vi "HostHoppingScan_v2_BoostedMultiRegion.vi"() -> ()   [LabVIEW 2024]
uses:
  <vilib>/Analysis/6fits.llb/Curve Fitting Criteria.ctl
  <vilib>/FPGAPlugInAG/USB-7845R OEM/niLvFpga_Open_USB-7845R OEM.vi
  <vilib>/rvi/interface/common/dynamic/niFpgaDynamicAddResources.vi
  <vilib>/Utility/error.llb/Error Cluster From Error Code.vi
  <vilib>/rvi/errors/niLvFpgaAdjustHostInterfaceError.vi
  <vilib>/rvi/interface/common/niFpgaWaitOnOcc.vi
  <vilib>/FPGAPlugInAG/Dynamic/niLvFpga_Close_Dynamic.vi
  <vilib>/rvi/interface/nirviOpenFPGA/nirviOpenFPGA.xnode
  FPGA Bitfiles/hoppingsicmv2_FPGATarget_FPGAHoppingScanB_lvkcmxVGkic.lvbitx
  <vilib>/rvi/interface/nirviMethod/nirviMethod.xnode
  <vilib>/rvi/interface/nirviReadWriteControl/nirviReadWriteControl.xnode
  <vilib>/rvi/interface/nirviCloseFPGA/nirviCloseFPGA.xnode
  NiFpgaLv.dll
  <vilib>/rvi/interface/Simulation/niFpgaSimulationCallBeginRW.vi
  <vilib>/rvi/errors/niLvFpgaMergeErrorWithErrorCode.vi
  <vilib>/FPGAPlugInAG/Dynamic/niLvFpga_ReadFifo_Dynamic.vi
  <vilib>/FPGAPlugInAG/Dynamic/niLvFpga_WriteFifo_Dynamic.vi
  <vilib>/Analysis/NI_AALPro.lvlib
  <vilib>/FPGAPlugInAG/Dynamic/niLvFpga_ConfigureFifo_Dynamic.vi
panel:
  out "RegionScanning":string
  in  "Auto Image \nSegmentation?":bool
  out "Adapted_YOffset um":dbl format="%#_13g"
  out "Adapted_XOffset um":dbl format="%#_13g"
  out "Adapted_YNum":i32
  out "Adapted_XNum":i32
  in  "Scanning Settings":T1(tab)
  in  "Retract (edge) um":dbl format="%#_13g"
  in  "FrameNum":u32
  in  "XNum":i32
  in  "YNum":i32
  in  "FF_Threshold %":dbl format="%#_13g"
  in  "XStepSize um":dbl format="%#_13g"
  in  "YStepSize um":dbl format="%#_13g"
  in  "YOffset um":dbl format="%#_13g"
  in  "XOffset um":dbl format="%#_13g"
  in  "Retract (flat) um":dbl format="%#_13g"
  in  "RetRate um/s":dbl format="%#_13g"
  in  "FF_AppRate um/s":dbl format="%#_13g"
  in  "NF_AppRate um/s":dbl format="%#_13g"
  in  "Pressure kPa":dbl format="%#_13g"
  in  "NF_Threshold %":dbl format="%#_13g"
  in  "Turning Distance um":dbl format="%#_13g"
  in  "CoordCalThreshold %":dbl format="%#_13g"
  in  "CoordCalRetract um":dbl format="%#_13g"
  in  "YCoordCalEnd um":dbl format="%#_13g"
  in  "XCoordCalEnd um":dbl format="%#_13g"
  in  "YCoordCalBegin um":dbl format="%#_13g"
  in  "XCoordCalBegin um":dbl format="%#_13g"
  in  "CoordCalAppRate um/s":dbl format="%#_13g"
  in  "CoordCalRetRate um/s":dbl format="%#_13g"
  in  "ScanMode":i32(knob) min=0 max=3 scale=0.0..3.0
  out "Signal Size":i32
  out "Done?":bool
  out "HTT_Buffer_Write":u32
  out "Scanned Points":i32
  in  "stop":bool
  in  "Notes":string
  in  "GraphTab":T2(tab)
  out "Topography":dbl[][](graph)
  out "Retract Map":dbl[][](graph)
  out "IZCurve":cluster{dbl[], dbl[]}(graph)
  out "Pressure Slope Map":dbl[][](graph)
  out "FPGA_Host_Buf_Depth":u32
  # "Calibrated Scan\n(New Calibration)"
  # "Calibrated Scan\n(Last Calibration)"
  # "Normal Scan"
  # "Background\nSubstrate Scan"
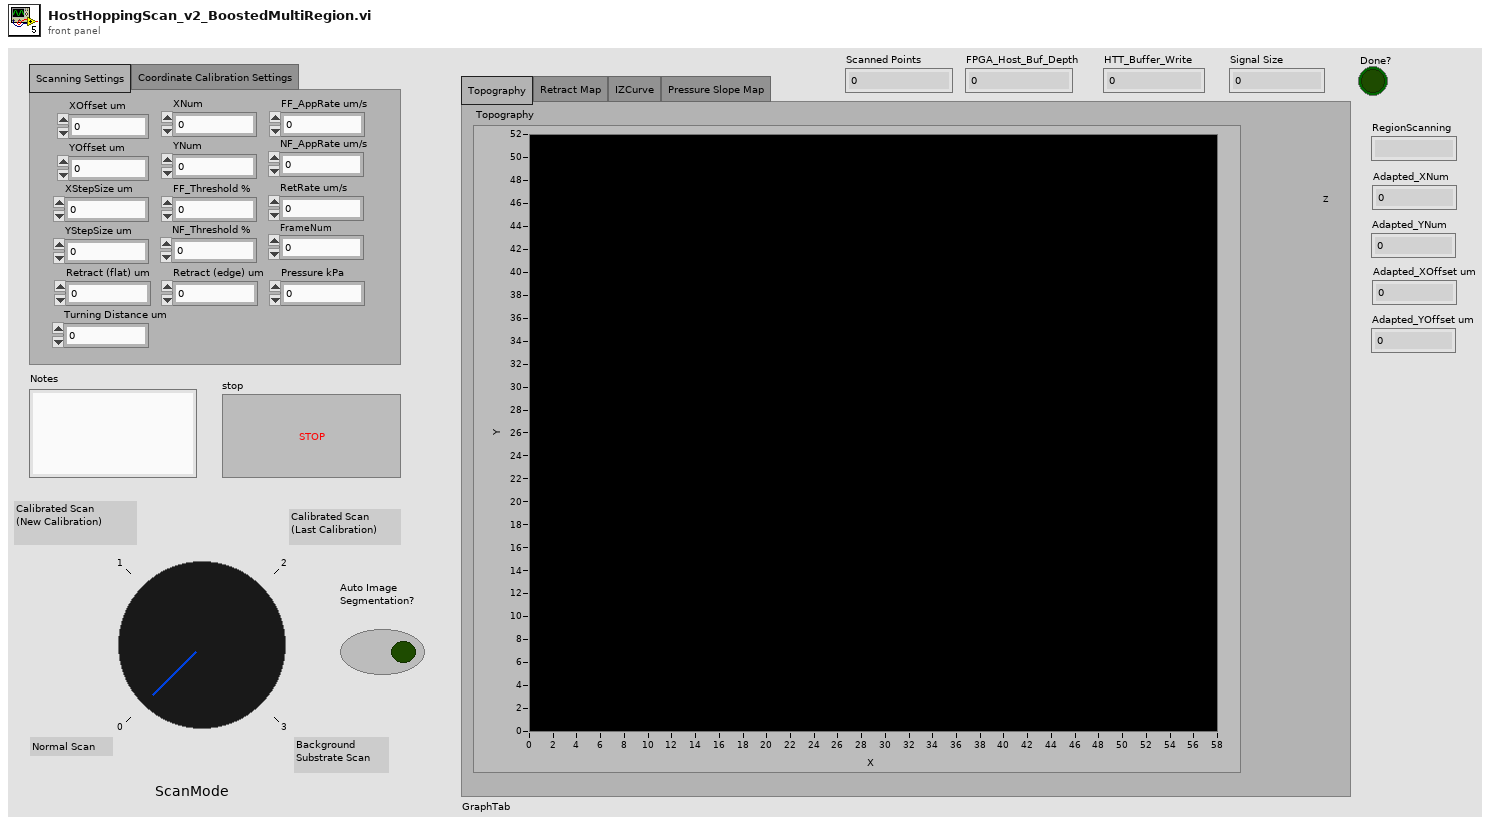
[diagram p1: front panel]
types:
  T1 = enum32{"Scanning Settings", "Coordinate Calibration Settings"}
  T2 = enum32{"Topography", "Retract Map", "IZCurve", "Pressure Slope Map"}
  T3 = typedef "NI_AALPro.lvlib/Curve Fitting Criteria.ctl" = u16
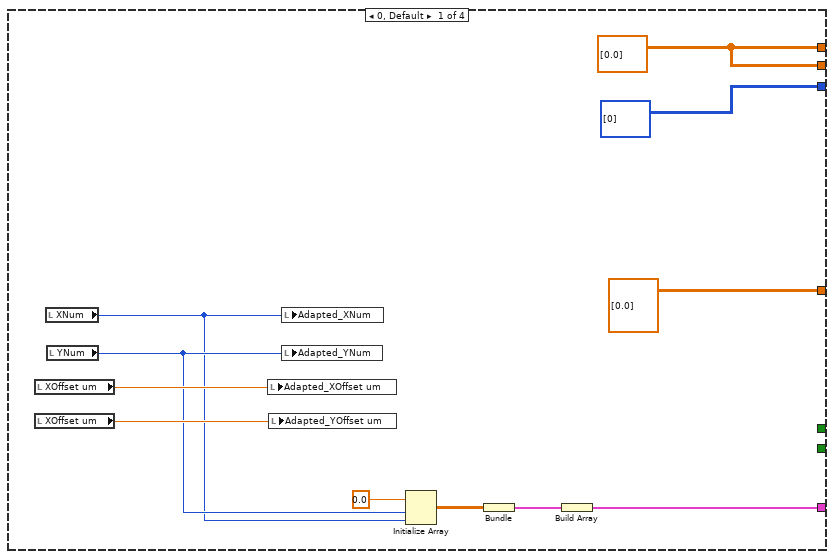
[diagram p3: hidden frame]
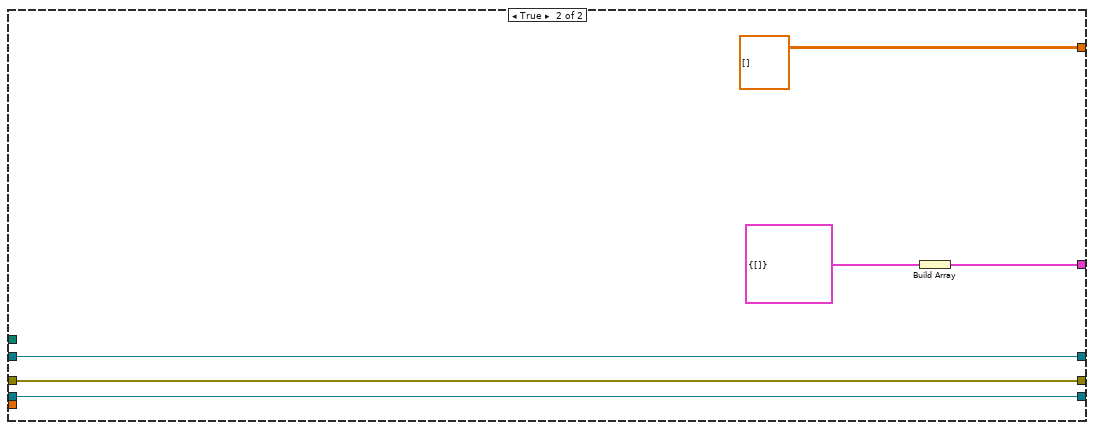
[diagram p4: hidden frame]
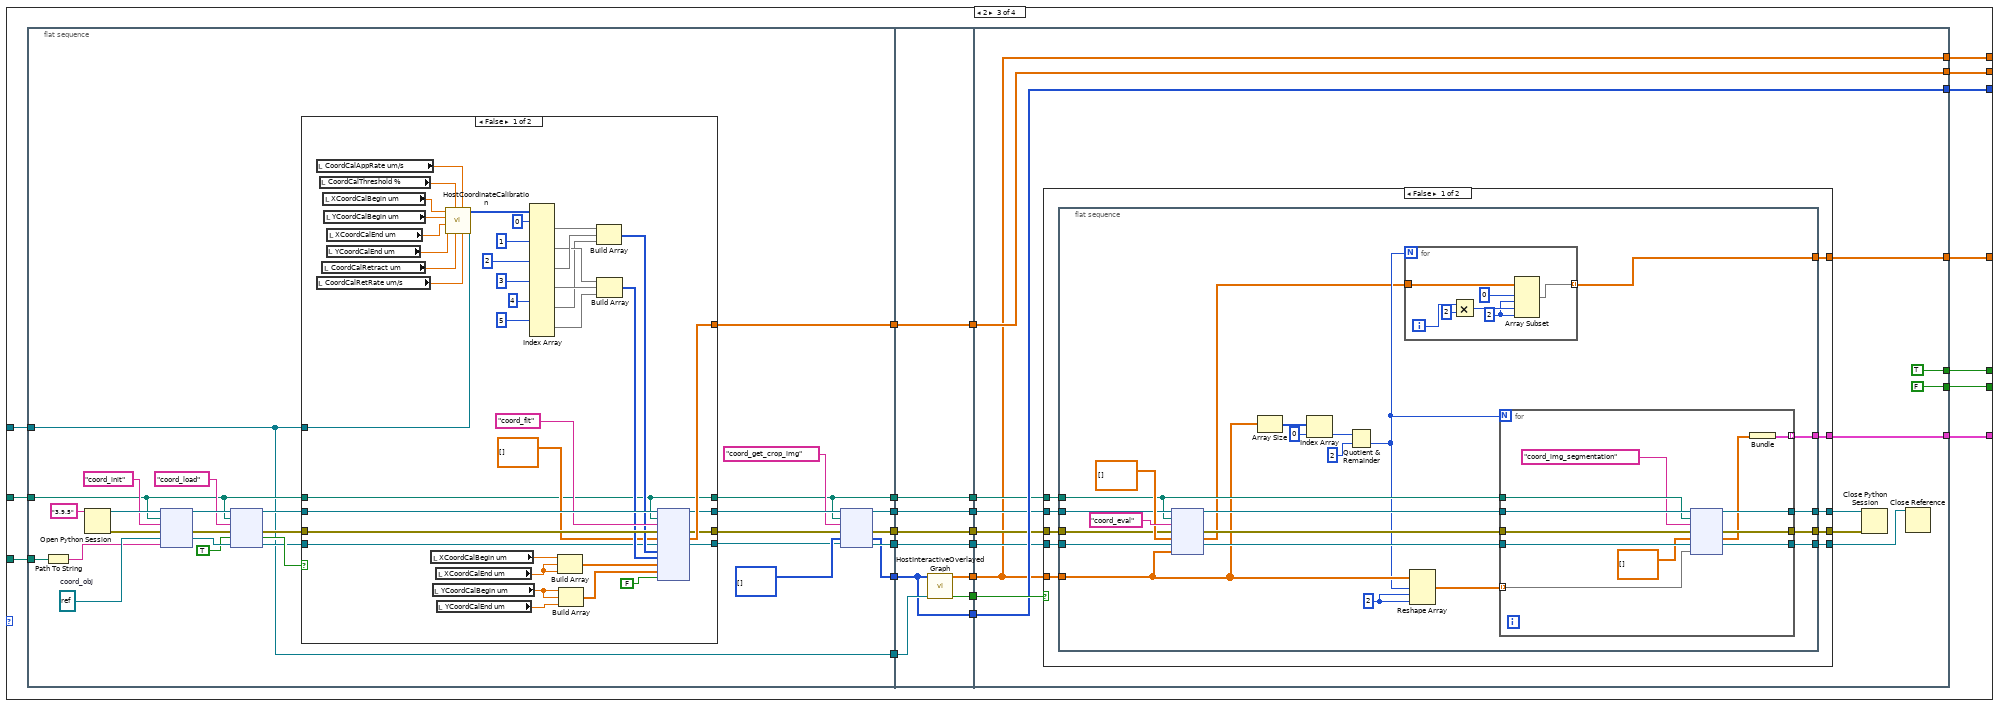
[diagram p5: hidden frame]
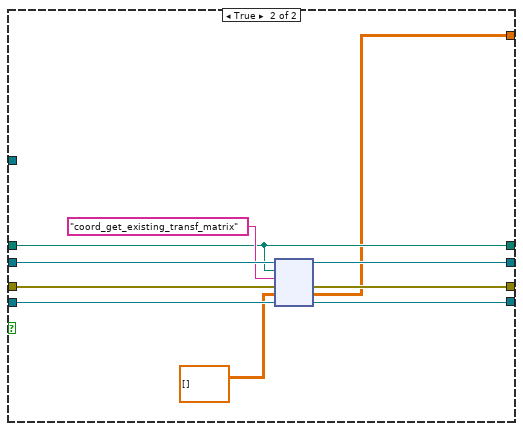
[diagram p6: hidden frame]
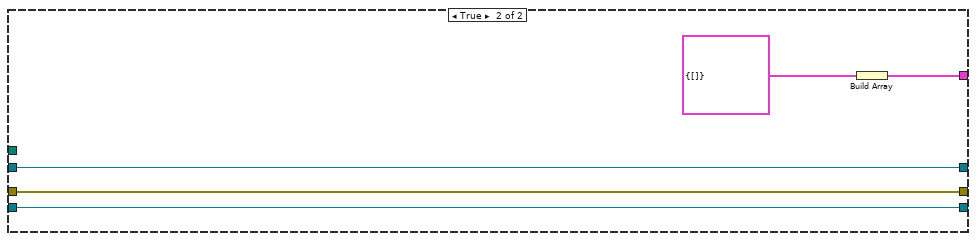
[diagram p7: hidden frame]
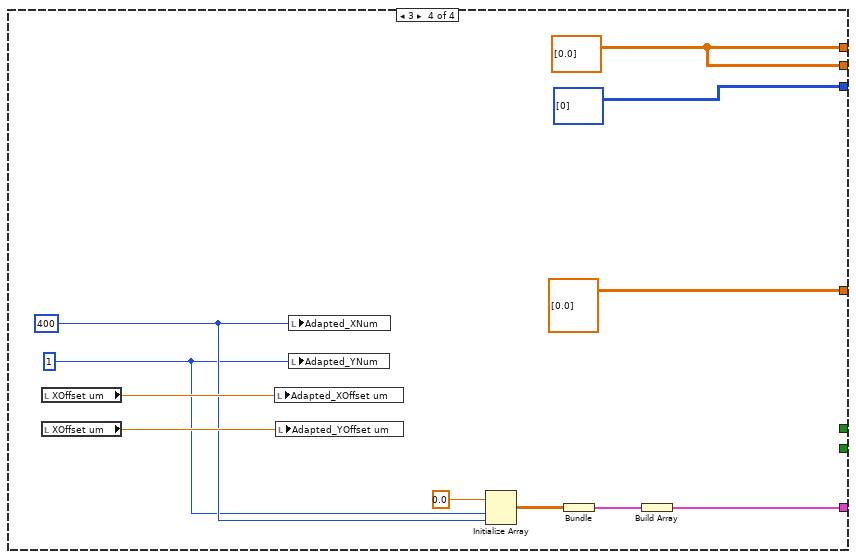
[diagram p8: hidden frame]
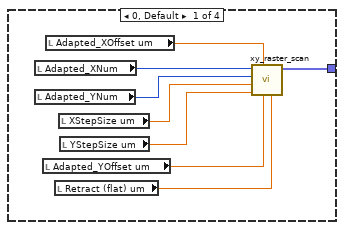
[diagram p14: hidden frame]
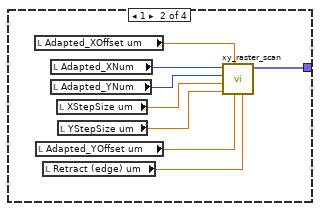
[diagram p15: hidden frame]
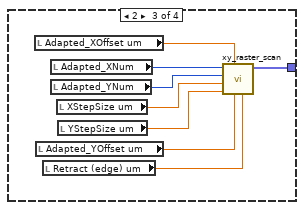
[diagram p16: hidden frame]
diagram:
  n1 = flat-sequence {
    tunnel: [w4] -> w2
    tunnel: w2 -> [w30]
    tunnel: [w27] -> w1
    tunnel: w1 -> [w1444]
    frame #0 {
      n2 = Obtain Queue(max queue size (-1, unlimited)=64, name (unnamed)="stop_sign", element data type=FALSE) -> (queue out=w4:refnum<queue>)  [unwired: 2 in, 2 out]
    }
    frame #1 {
      n3 = flat-sequence {
        tunnel: [w52] -> w31
        tunnel: w30 -> [w52]
        tunnel: w31 -> [w58]
        tunnel: [w58] -> w25
        tunnel: [w54] -> w24
        tunnel: [w107] -> w22
        tunnel: [w108] -> w21
        tunnel: [w109] -> w20
        tunnel: [w110] -> w19
        tunnel: [w111] -> w18
        tunnel: [w74] -> w17
        tunnel: w24 -> [w92]
        tunnel: w25 -> [w74]
        tunnel: [w72] -> w16
        tunnel: [w499] -> w39
        tunnel: [w497] -> w38
        tunnel: [w496] -> w37
        tunnel: [w498] -> w36
        tunnel: [w501] -> w29
        tunnel: w22 -> [w496]
        tunnel: w21 -> [w497]
        tunnel: w20 -> [w499]
        tunnel: w19 -> [w498]
        tunnel: w18 -> [w490]
        tunnel: [w490] -> w23
        tunnel: w17 -> [w494]
        tunnel: w16 -> [w491]
        tunnel: [w491] -> w15
        tunnel: [w489] -> w14
        tunnel: w39 -> [w526]
        tunnel: w38 -> [w525]
        tunnel: w37 -> [w524]
        tunnel: [w522] -> w35
        tunnel: [w521] -> w34
        tunnel: [w520] -> w33
        tunnel: [w519] -> w32
        tunnel: w36 -> [w523]
        tunnel: w29 -> [w518]
        tunnel: [w517] -> w28
        tunnel: w23 -> [w516]
        tunnel: w15 -> [w515]
        tunnel: w14 -> [w514]
        tunnel: [w514] -> w13
        tunnel: [w513] -> w12
        tunnel: [w512] -> w11
        tunnel: [w511] -> w10
        tunnel: [w510] -> w9
        tunnel: [w509] -> w8
        tunnel: [w508] -> w7
        tunnel: w35 -> [w1430]
        tunnel: w34 -> [w1436]
        tunnel: w33 -> [w1435]
        tunnel: w32 -> [w1434]
        tunnel: w28 -> [w1428]
        tunnel: [w1428] -> w26
        tunnel: w13 -> [w1418]
        tunnel: w12 -> [w1417]
        tunnel: w11 -> [w1416]
        tunnel: w10 -> [w1415]
        tunnel: w9 -> [w1414]
        tunnel: w8 -> [w1413]
        tunnel: w7 -> [w1412]
        tunnel: [w1443] -> w27
        tunnel: w26 -> [w1443]
        frame #0 {
          n4 = Wait (ms)(milliseconds to wait=u32 100) -> ()  [unwired: 1 out]
          "Done?" <- FALSE ("Done?")
          "Adapted_XNum" <- "XNum"
          "Adapted_YNum" <- "YNum"
          "Adapted_XOffset um" <- "XStepSize um"
          "Adapted_YOffset um" <- "YStepSize um"
        }
        frame #1 {
          n5 = call "File Dialog"("prompt"="Choose a path to save scanning image data files") -> ("selected path"=w54:path, "cancelled"=w56:bool, "error out"=w55:errorcluster)  [unwired: 11 in, 1 out]
          n6 = Stop(stop? (T)=w56) -> ()
          n7 = call <vilib>:"Clear Errors.vi"("error in (no error)"=w55) -> ()  [unwired: 5 in, 2 out]
        }
        frame #2 {
          w73 = refnum<k38> refnum  # db_obj
          # "coordinate calibration"
          # "use python to save data this time"
          n8 = Path To String(path=w92) -> (string=w106:string)
          n9 = local read "ScanMode"() -> (w75:i32)
          n10 = Get Queue Status(queue=w74) -> (# elements in queue=w91:i32)  [unwired: 2 in, 7 out]
          n11 = Concatenate Strings(w106, "_data.db" ("string")) -> (w105:string)
          n12 = Current VI's Path() -> (path=w97:path)
          n13 = Less Or Equal To 0?(x=w91) -> (x <= 0?=w90:bool)
          n14 = String To Path(string=w105) -> (path=w103:path)
          n15 = Strip Path(path=w97) -> (stripped path=w85:path)  [unwired: 1 out]
          n16 = call <vilib>:"Check if File or Folder Exists.vi"("path"=w103) -> ("file or folder exists?"=w104:bool)  [unwired: 8 in, 2 out]
          n17 = Build Path(base path=w85, name or relative path=path "py/coord_transform.py") -> (appended path=w87:path)
          n18 = Build Path(base path=w85, name or relative path=path "coordinate_calibration/tmp_calibrated_coord") -> (appended path=w84:path)
          n19 = Select(t=w75, s=w90, f=0 ("t")) -> (s? t:f=w89:i32)
          n20 = Build Path(base path=w85, name or relative path=path "py/data_db_arrangement_boosted_multi_region.py") -> (appended path=w110:path)
          n21 = case shown="1" w89 {
            tunnel: w87 -> [_ w145 w313 _]
            tunnel: w84 -> [_ w147 w312 _]
            tunnel: w74 -> [_ w146 w311 _]
            tunnel: [w120 w144 w290 w477] -> w111
            tunnel: [i32[][] [[0]] w143 w292 i32[][] [[0]]] -> w60
            tunnel: [w119 w142 w291 w485] -> w61
            tunnel: [w119 w141 w293 w485] -> w62
            tunnel: [_ w140 w294 _] -> w63
            tunnel: [_ w139 w295 _] -> w64
            tunnel: [dbl[][][] [[[0.0]]] ("OutputRetractMap um") w123 w289 dbl[][][] [[[0.0]]] ("OutputRetractMap um")] -> w72
            frame 0, Default {
              w119 = dbl[][] [[0.0]] ("Output_Coord")
              n22 = local read "XOffset um"() -> (w122:dbl)
              n23 = local read "XOffset um"() -> (w121:dbl)
              n24 = local read "XNum"() -> (w112:i32)
              n25 = local read "YNum"() -> (w113:i32)
              n26 = local write "Adapted_XOffset um"(w122) -> ()
              n27 = local write "Adapted_YOffset um"(w121) -> ()
              n28 = local write "Adapted_XNum"(w112) -> ()
              n29 = local write "Adapted_YNum"(w113) -> ()
              n30 = Initialize Array(0.0, w113, w112) -> (w115:dbl[][])
              n31 = Bundle(w115) -> (w114:cluster{dbl[][]})  [unwired: 1 in]
              n32 = Build Array(w114) -> (w120:cluster{dbl[][]}[])
            }
            frame 1 {
              n33 = flat-sequence {
                tunnel: w147 -> [w196]
                tunnel: w146 -> [w149]
                tunnel: w145 -> [w152]
                tunnel: [w152] -> w129
                tunnel: [w160] -> w131
                tunnel: [w155] -> w133
                tunnel: [w154] -> w135
                tunnel: [w153] -> w136
                tunnel: [w150] -> w138
                tunnel: [w149] -> w127
                tunnel: w138 -> [w210]
                tunnel: [w210] -> w137
                tunnel: w136 -> [w202]
                tunnel: w135 -> [w209]
                tunnel: [w209] -> w134
                tunnel: w133 -> [w208]
                tunnel: [w208] -> w132
                tunnel: w131 -> [w207]
                tunnel: [w207] -> w130
                tunnel: w129 -> [w206]
                tunnel: [w206] -> w128
                tunnel: w127 -> [w205]
                tunnel: [w204] -> w126
                tunnel: [w203] -> w125
                tunnel: [w202] -> w124
                tunnel: [w222] -> w144
                tunnel: [w212] -> w143
                tunnel: [w214] -> w142
                tunnel: [w221] -> w141
                tunnel: [TRUE] -> w140
                tunnel: [FALSE] -> w139
                tunnel: w137 -> [w221]
                tunnel: w134 -> [w216]
                tunnel: w132 -> [w217]
                tunnel: w130 -> [w218]
                tunnel: w128 -> [w215]
                tunnel: w126 -> [w214]
                tunnel: w125 -> [w213]
                tunnel: w124 -> [w212]
                tunnel: [w211] -> w123
                frame #0 {
                  w197 = refnum<k38> refnum  # coord_obj
                  # "extended img bundle"
                  # "retracted img bundle"
                  n34 = Path To String(path=w196) -> (string=w195:string)
                  n35 = local read "CoordCalAppRate um/s"() -> (w189:dbl)
                  n36 = local read "CoordCalRetRate um/s"() -> (w187:dbl)
                  n37 = local read "CoordCalThreshold %"() -> (w190:dbl)
                  n38 = local read "CoordCalRetract um"() -> (w188:dbl)
                  n39 = local read "XCoordCalBegin um"() -> (w194:dbl)
                  n40 = local read "YCoordCalBegin um"() -> (w193:dbl)
                  n41 = local read "YCoordCalEnd um"() -> (w191:dbl)
                  n42 = local read "XCoordCalEnd um"() -> (w192:dbl)
                  n43 = Open Python Session(python version="3.9.5" ("Python version")) -> (session out=w200:refnum<k35>, error out=w199:errorcluster)  [unwired: 2 in]
                  n44 = node(w200, w152, "coord_init" ("Python version"), w199, w197, w195) -> (w174:refnum<k35>, w172:errorcluster, w173:refnum<k38>)  [unwired: 1 in, 2 out]
                  n45 = call "HostCoordinateCalibration.vi"("stop_sign_queue"=w149, "RetRate um/s"=w187, "AppRate um/s"=w189, "Retract um"=w188, "Threshold %"=w190, "YCalibrationEnd um"=w191, "XCalibrationEnd um"=w192, "YCalibrationOffset um"=w193, "XCalibrationOffset um"=w194) -> ("img_bundle"=w186:i32[][][])  [unwired: 2 in]
                  n46 = local read "XCoordCalBegin um"() -> (w169:dbl)
                  n47 = local read "YCoordCalBegin um"() -> (w166:dbl)
                  n48 = local read "XCoordCalEnd um"() -> (w168:dbl)
                  n49 = local read "YCoordCalEnd um"() -> (w167:dbl)
                  n50 = Index Array(array=w186, index (dim 0) #1=0 ("index (page)"), index (dim 0) #2=1 ("index (page)"), index (dim 0) #3=2 ("index (page)"), index (dim 0) #4=3 ("index (page)"), index (dim 0) #5=4 ("index (page)"), index (dim 0) #6=5 ("index (page)")) -> (element #1=w148:i32[][], element #2=w178:i32[][], element #3=w179:i32[][], element #4=w177:i32[][], element #5=w176:i32[][], element #6=w175:i32[][])  [unwired: 12 in]
                  n51 = Build Array(w169, w168, w168) -> (w165:dbl[])
                  n52 = Build Array(w166, w166, w167) -> (w164:dbl[])
                  n53 = Build Array(w148, w179, w176) -> (w171:i32[][][])
                  n54 = Build Array(w178, w177, w175) -> (w170:i32[][][])
                  n55 = node(w174, w152, "coord_fit" ("function name"), w172, dbl[][] [], w173, w171, w170, w165, w164, TRUE) -> (w161:refnum<k35>, w159:errorcluster, w150:dbl[][], w157:refnum<k38>)  [unwired: 5 in, 2 out]
                  n56 = node(w161, w152, "coord_get_crop_img" ("function name"), w159, i32[][] [], w157) -> (w160:refnum<k35>, w155:errorcluster, w153:i32[][], w154:refnum<k38>)  [unwired: 2 out]
                }
                frame #1 {
                  n57 = call "HostInteractiveOverlayedGraph.vi"("stop_sign_queue"=w205, "InputImg"=w202) -> ("Break"=w203:bool, "Output_Coord"=w204:dbl[][])  [unwired: 8 in]
                }
                frame #2 {
                  n58 = case shown="False" w213 {
                    tunnel: [w235 w288] -> w225
                    tunnel: [w234 w287] -> w224
                    tunnel: [w233 w286] -> w223
                    tunnel: [w227 w283] -> w222
                    tunnel: w214 -> [w232 _]
                    tunnel: w218 -> [w231 w288]
                    tunnel: w217 -> [w230 w287]
                    tunnel: w216 -> [w229 w286]
                    tunnel: w215 -> [w228 _]
                    tunnel: [w226 dbl[][][] [] ("OutputRetractMap um")] -> w211
                    frame False {
                      n59 = flat-sequence {
                        tunnel: [w245] -> w227
                        tunnel: [w255] -> w233
                        tunnel: [w256] -> w234
                        tunnel: [w257] -> w235
                        tunnel: w228 -> [w246]
                        tunnel: w229 -> [w252]
                        tunnel: w230 -> [w253]
                        tunnel: w231 -> [w254]
                        tunnel: w232 -> [w237]
                        tunnel: [w239] -> w226
                        frame #0 {
                          n60 = node(w254, w246, "coord_eval" ("function name"), w253, dbl[][] [], w252, w237) -> (w249:refnum<k35>, w248:errorcluster, w240:dbl[][], w247:refnum<k38>)  [unwired: 1 in, 2 out]
                          n61 = Array Size(array=w237) -> (size(s)=w244:i32[])
                          n62 = Index Array(array=w244, index=0) -> (element=w242:i32)
                          n63 = Quotient & Remainder(x=w242, y=2 ("index")) -> (floor(x/y)=w238:i32)  [unwired: 1 out]
                          n64 = for {
                            N: w238 -> [_]
                            tunnel: w237 -> [w263]
                            tunnel: [w258] -> w236 mode=indexing
                            i -> [w262]
                            n65 = Multiply(x=w262, y=2) -> (x*y=w260:i32)
                            n66 = Array Subset(array=w263, index (row)=w260, length (row)=2 ("length")) -> (w258:dbl[][])  [unwired: 2 in]
                          }
                          n67 = for {
                            N: w238 -> [_]
                            tunnel: w240 -> [w267]
                            tunnel: [w266] -> w239 mode=indexing
                            i -> [w264]
                            w268 = 2 ("length")
                            n68 = Multiply(x=2 ("y"), y=w264) -> (x*y=w270:i32)
                            n69 = Array Subset(array=w267, index (row)=0 ("index"), length (row)=w268, index (col)=w270, length (col)=w268) -> (w266:dbl[][])
                          }
                          n70 = for {
                            N: w238 -> [_]
                            tunnel: w236 -> [w279] mode=indexing
                            tunnel: w246 -> [w273]
                            tunnel: [w271] -> w245 mode=indexing
                            tunnel: w249 -> [w278]
                            tunnel: [w282] -> w257
                            tunnel: w248 -> [w277]
                            tunnel: [w281] -> w256
                            tunnel: w247 -> [w276]
                            tunnel: [w280] -> w255
                            n71 = node(w278, w273, "coord_img_segmentation" ("function name"), w277, dbl[][] [], w276, w279) -> (w282:refnum<k35>, w281:errorcluster, w272:dbl[][], w280:refnum<k38>)  [unwired: 1 in, 2 out]
                            n72 = Bundle(w272) -> (w271:cluster{dbl[][]})  [unwired: 1 in]
                          }
                        }
                      }
                    }
                    frame True {
                      n73 = Build Array(cluster{dbl[][]} {[]}) -> (w283:cluster{dbl[][]}[])
                    }
                  }
                  n74 = Close Python Session(session in=w225, error in=w224) -> ()  [unwired: 1 out]
                  n75 = Close Reference(reference=w223) -> ()  [unwired: 1 in, 1 out]
                }
              }
            }
            frame 2 {
              n76 = flat-sequence {
                tunnel: w313 -> [w327]
                tunnel: w312 -> [w336]
                tunnel: w311 -> [w325]
                tunnel: [w314] -> w310
                tunnel: [w325] -> w309
                tunnel: [w324] -> w308
                tunnel: [w318] -> w305
                tunnel: [w317] -> w303
                tunnel: [w316] -> w301
                tunnel: [w315] -> w299
                tunnel: w310 -> [w394]
                tunnel: w309 -> [w402]
                tunnel: w308 -> [w401]
                tunnel: [w401] -> w307
                tunnel: [w400] -> w306
                tunnel: w305 -> [w400]
                tunnel: [w399] -> w304
                tunnel: w303 -> [w399]
                tunnel: [w398] -> w302
                tunnel: w301 -> [w398]
                tunnel: [w397] -> w300
                tunnel: w299 -> [w397]
                tunnel: [w396] -> w298
                tunnel: [w395] -> w297
                tunnel: [w394] -> w296
                tunnel: w307 -> [w414]
                tunnel: w306 -> [w412]
                tunnel: w304 -> [w411]
                tunnel: w302 -> [w410]
                tunnel: w300 -> [w409]
                tunnel: w298 -> [w408]
                tunnel: w297 -> [w417]
                tunnel: w296 -> [w413]
                tunnel: [FALSE] -> w295
                tunnel: [TRUE] -> w294
                tunnel: [w414] -> w293
                tunnel: [w413] -> w292
                tunnel: [w408] -> w291
                tunnel: [w404] -> w290
                tunnel: [w403] -> w289
                frame #0 {
                  w338 = refnum<k38> refnum  # coord_obj
                  n77 = Path To String(path=w336) -> (string=w337:string)
                  n78 = Open Python Session(python version="3.9.5" ("Python version")) -> (session out=w341:refnum<k35>, error out=w340:errorcluster)  [unwired: 2 in]
                  n79 = node(w341, w327, "coord_init" ("Python version"), w340, w338, w337) -> (w335:refnum<k35>, w334:errorcluster, w333:refnum<k38>)  [unwired: 1 in, 2 out]
                  n80 = node(w335, w327, "coord_load" ("Python version"), w334, TRUE, w333) -> (w329:refnum<k35>, w328:errorcluster, w330:bool, w326:refnum<k38>)  [unwired: 2 out]
                  n81 = case shown="False" w330 {
                    tunnel: w329 -> [w361 w393]
                    tunnel: w328 -> [w359 w392]
                    tunnel: w325 -> [w375 _]
                    tunnel: w327 -> [w343 w385]
                    tunnel: w326 -> [w349 w391]
                    tunnel: [w347 w384] -> w324
                    tunnel: [w346 w388] -> w323
                    tunnel: [w345 w387] -> w320
                    tunnel: [w344 w386] -> w319
                    tunnel: [w343 w385] -> w318
                    frame False {
                      n82 = local read "CoordCalAppRate um/s"() -> (w378:dbl)
                      n83 = local read "CoordCalRetRate um/s"() -> (w376:dbl)
                      n84 = local read "CoordCalThreshold %"() -> (w379:dbl)
                      n85 = local read "CoordCalRetract um"() -> (w377:dbl)
                      n86 = local read "XCoordCalBegin um"() -> (w383:dbl)
                      n87 = local read "YCoordCalBegin um"() -> (w382:dbl)
                      n88 = local read "YCoordCalEnd um"() -> (w380:dbl)
                      n89 = local read "XCoordCalEnd um"() -> (w381:dbl)
                      n90 = local read "XCoordCalBegin um"() -> (w358:dbl)
                      n91 = local read "YCoordCalBegin um"() -> (w355:dbl)
                      n92 = local read "XCoordCalEnd um"() -> (w357:dbl)
                      n93 = local read "YCoordCalEnd um"() -> (w356:dbl)
                      n94 = call "HostCoordinateCalibration.vi"("stop_sign_queue"=w375, "RetRate um/s"=w376, "AppRate um/s"=w378, "Retract um"=w377, "Threshold %"=w379, "YCalibrationEnd um"=w380, "XCalibrationEnd um"=w381, "YCalibrationOffset um"=w382, "XCalibrationOffset um"=w383) -> ("img_bundle"=w362:i32[][][])  [unwired: 2 in]
                      n95 = Index Array(array=w362, index (dim 0) #1=0 ("index (page)"), index (dim 0) #2=1 ("index (page)"), index (dim 0) #3=2 ("index (page)"), index (dim 0) #4=3 ("index (page)"), index (dim 0) #5=4 ("index (page)"), index (dim 0) #6=5 ("index (page)")) -> (element #1=w363:i32[][], element #2=w367:i32[][], element #3=w368:i32[][], element #4=w366:i32[][], element #5=w365:i32[][], element #6=w364:i32[][])  [unwired: 12 in]
                      n96 = Build Array(w358, w357, w357) -> (w352:dbl[])
                      n97 = Build Array(w355, w355, w356) -> (w351:dbl[])
                      n98 = Build Array(w363, w368, w365) -> (w354:i32[][][])
                      n99 = Build Array(w367, w366, w364) -> (w353:i32[][][])
                      n100 = node(w361, w343, "coord_fit" ("function name"), w359, dbl[][] [], w349, w354, w353, w352, w351, FALSE) -> (w346:refnum<k35>, w345:errorcluster, w347:dbl[][], w344:refnum<k38>)  [unwired: 5 in, 2 out]
                    }
                    frame True {
                      n101 = node(w393, w385, "coord_get_existing_transf_matrix" ("Python version"), w392, dbl[][] [], w391) -> (w388:refnum<k35>, w387:errorcluster, w384:dbl[][], w386:refnum<k38>)  [unwired: 2 out]
                    }
                  }
                  n102 = node(w323, w318, "coord_get_crop_img" ("function name"), w320, i32[][] [], w319) -> (w317:refnum<k35>, w316:errorcluster, w314:i32[][], w315:refnum<k38>)  [unwired: 2 out]
                }
                frame #1 {
                  n103 = call "HostInteractiveOverlayedGraph.vi"("stop_sign_queue"=w402, "InputImg"=w394) -> ("Break"=w395:bool, "Output_Coord"=w396:dbl[][])  [unwired: 8 in]
                }
                frame #2 {
                  n104 = case shown="False" w417 {
                    tunnel: w412 -> [w427 _]
                    tunnel: w411 -> [w426 w474]
                    tunnel: w410 -> [w425 w473]
                    tunnel: w409 -> [w424 w472]
                    tunnel: w408 -> [w423 _]
                    tunnel: [w422 w474] -> w407
                    tunnel: [w421 w473] -> w406
                    tunnel: [w420 w472] -> w405
                    tunnel: [w419 w470] -> w404
                    tunnel: [w418 _] -> w403
                    frame False {
                      n105 = flat-sequence {
                        tunnel: [w450] -> w422
                        tunnel: [w449] -> w421
                        tunnel: [w448] -> w420
                        tunnel: [w447] -> w419
                        tunnel: w423 -> [w432]
                        tunnel: w424 -> [w442]
                        tunnel: w425 -> [w443]
                        tunnel: w426 -> [w444]
                        tunnel: w427 -> [w438]
                        tunnel: [w429] -> w418
                        frame #0 {
                          w433 = 2 ("index")
                          n106 = node(w444, w438, "coord_eval" ("function name"), w443, dbl[][] [], w442, w432) -> (w441:refnum<k35>, w440:errorcluster, w428:dbl[][], w439:refnum<k38>)  [unwired: 1 in, 2 out]
                          n107 = Array Size(array=w432) -> (size(s)=w437:i32[])
                          n108 = Index Array(array=w437, index=0) -> (element=w435:i32)
                          n109 = Quotient & Remainder(x=w435, y=2 ("index")) -> (floor(x/y)=w430:i32)  [unwired: 1 out]
                          n110 = for {
                            N: w430 -> [_]
                            tunnel: w428 -> [w457]
                            tunnel: [w454] -> w429 mode=indexing
                            i -> [w456]
                            w451 = 2 ("length")
                            n111 = Multiply(x=w456, y=2) -> (x*y=w453:i32)
                            n112 = Array Subset(array=w457, index (row)=0 ("index"), length (row)=w451, index (col)=w453, length (col)=w451) -> (w454:dbl[][])
                          }
                          n113 = Reshape Array(w432, w430, w433, w433) -> (w431:dbl[][][])
                          n114 = for {
                            N: w430 -> [_]
                            tunnel: w431 -> [w466] mode=indexing
                            tunnel: w438 -> [w465]
                            tunnel: [w458] -> w447 mode=indexing
                            tunnel: w441 -> [w469]
                            tunnel: [w464] -> w450
                            tunnel: w440 -> [w468]
                            tunnel: [w462] -> w449
                            tunnel: w439 -> [w467]
                            tunnel: [w461] -> w448
                            n115 = node(w469, w465, "coord_img_segmentation" ("function name"), w468, dbl[][] [], w467, w466) -> (w464:refnum<k35>, w462:errorcluster, w459:dbl[][], w461:refnum<k38>)  [unwired: 1 in, 2 out]
                            n116 = Bundle(w459) -> (w458:cluster{dbl[][]})  [unwired: 1 in]
                          }
                        }
                      }
                    }
                    frame True {
                      n117 = Build Array(cluster{dbl[][]} {[]}) -> (w470:cluster{dbl[][]}[])
                    }
                  }
                  n118 = Close Python Session(session in=w407, error in=w406) -> ()  [unwired: 1 out]
                  n119 = Close Reference(reference=w405) -> ()  [unwired: 1 in, 1 out]
                }
              }
            }
            frame 3 {
              w475 = 1 ("Adapted_XNum")
              w476 = 400 ("Adapted_XNum")
              w485 = dbl[][] [[0.0]] ("Output_Coord")
              n120 = local read "XOffset um"() -> (w482:dbl)
              n121 = local read "XOffset um"() -> (w481:dbl)
              n122 = local write "Adapted_XOffset um"(w482) -> ()
              n123 = local write "Adapted_YOffset um"(w481) -> ()
              n124 = local write "Adapted_XNum"(w476) -> ()
              n125 = local write "Adapted_YNum"(w475) -> ()
              n126 = Initialize Array(0.0, w475, w476) -> (w479:dbl[][])
              n127 = Bundle(w479) -> (w478:cluster{dbl[][]})  [unwired: 1 in]
              n128 = Build Array(w478) -> (w477:cluster{dbl[][]}[])
            }
          }
          n129 = case shown="True" w104 {
            tunnel: w103 -> [w486 w488]
            tunnel: [w486 w487] -> w102
            frame False {
            }
            frame True {
              n130 = Delete(path (use dialog)=w488) -> (deleted path=w487:path)  [unwired: 4 in, 2 out]
            }
          }
          n131 = Path To String(path=w102) -> (string=w94:string)
          n132 = Open Python Session(python version="3.9.5" ("Python version")) -> (session out=w99:refnum<k35>, error out=w98:errorcluster)  [unwired: 2 in]
          n133 = node(w99, w110, "db_init" ("Python version"), w98, w73, w94) -> (w83:refnum<k35>, w82:errorcluster, w81:refnum<k38>)  [unwired: 1 in, 2 out]
          n134 = local read "CoordCalAppRate um/s"() -> (w65:dbl)
          n135 = local read "CoordCalRetRate um/s"() -> (w59:dbl)
          n136 = local read "CoordCalThreshold %"() -> (w67:dbl)
          n137 = local read "CoordCalRetract um"() -> (w66:dbl)
          n138 = local read "XCoordCalBegin um"() -> (w71:dbl)
          n139 = local read "YCoordCalBegin um"() -> (w70:dbl)
          n140 = local read "YCoordCalEnd um"() -> (w68:dbl)
          n141 = local read "XCoordCalEnd um"() -> (w69:dbl)
          n142 = node(w83, w110, "db_insert_coordinate_calibration" ("function name"), w82, w81, w71, w70, w69, w68, w67, w66, w65, w59, w60, w61, w62, w63, w64) -> (w80:refnum<k35>, w79:errorcluster, w78:refnum<k38>)  [unwired: 15 in, 2 out]
          n143 = node(w80, w110, "db_start_global_timer" ("function name"), w79, w78) -> (w109:refnum<k35>, w108:errorcluster, w107:refnum<k38>)  [unwired: 2 in, 2 out]
        }
        frame #3 {
          n144 = Get Queue Status(queue=w494) -> (queue out=w493:refnum<queue>, # elements in queue=w495:i32)  [unwired: 2 in, 6 out]
          n145 = Greater Than 0?(x=w495) -> (x > 0?=w492:bool)
          n146 = case shown="True" w492 {
            tunnel: w493 -> [w502 w505]
            tunnel: [w502 w503] -> w501
            frame False {
            }
            frame True {
              n147 = flat-sequence {
                tunnel: w505 -> [w506]
                tunnel: [w506] -> w504
                tunnel: w504 -> [w507]
                tunnel: [w507] -> w503
                frame #0 {
                  n148 = Release Queue(queue=w506) -> ()  [unwired: 2 in, 3 out]
                }
                frame #1 {
                  n149 = Stop() -> ()  [unwired: 1 in]
                }
              }
            }
          }
          n150 = Array Size(array=w490) -> (size(s)=w489:i32)
          n151 = Wait (ms)(milliseconds to wait=u32 200) -> ()  [unwired: 1 out]
        }
        frame #4 {
          n152 = for {
            N: w514 -> [_]
            tunnel: w516 -> [w559] mode=indexing
            tunnel: w523 -> [w566]
            tunnel: [w565] -> w522
            tunnel: w526 -> [w569]
            tunnel: [w564] -> w521
            tunnel: w525 -> [w568]
            tunnel: [w563] -> w520
            tunnel: w524 -> [w567]
            tunnel: [w562] -> w519
            tunnel: w518 -> [w561]
            tunnel: [w560] -> w517
            tunnel: w515 -> [w545] mode=indexing
            tunnel: w514 -> [w541]
            tunnel: [w532] -> w513 mode=indexing
            tunnel: [w531] -> w512 mode=indexing
            tunnel: [w530] -> w511 mode=indexing
            tunnel: [w529] -> w510 mode=indexing
            tunnel: [w528] -> w509 mode=indexing
            tunnel: [w527] -> w508 mode=indexing
            i -> [w544]
            stop <- w546 stop-if-true
            n153 = flat-sequence {
              tunnel: w559 -> [w577]
              tunnel: w561 -> [w586]
              tunnel: w566 -> [w587]
              tunnel: w567 -> [w588]
              tunnel: w568 -> [w589]
              tunnel: w569 -> [w590]
              tunnel: [w590] -> w558
              tunnel: [w589] -> w556
              tunnel: [w588] -> w554
              tunnel: [w587] -> w552
              tunnel: [w586] -> w550
              tunnel: [w576] -> w548
              tunnel: w545 -> [w585]
              tunnel: w544 -> [w582]
              tunnel: [w582] -> w542
              tunnel: w541 -> [w584]
              tunnel: [w584] -> w539
              tunnel: w558 -> [w638]
              tunnel: [w638] -> w557
              tunnel: w556 -> [w637]
              tunnel: [w637] -> w555
              tunnel: w554 -> [w636]
              tunnel: [w636] -> w553
              tunnel: w552 -> [w635]
              tunnel: [w635] -> w551
              tunnel: w550 -> [w634]
              tunnel: [w634] -> w549
              tunnel: w548 -> [w629]
              tunnel: [w628] -> w547
              tunnel: [w627] -> w543
              tunnel: w542 -> [w627]
              tunnel: [w626] -> w540
              tunnel: w539 -> [w626]
              tunnel: w557 -> [w652]
              tunnel: w555 -> [w651]
              tunnel: w553 -> [w650]
              tunnel: w551 -> [w649]
              tunnel: w549 -> [w644]
              tunnel: w547 -> [w642]
              tunnel: w543 -> [w640]
              tunnel: w540 -> [w639]
              tunnel: [w648] -> w538
              tunnel: [w647] -> w537
              tunnel: [w646] -> w536
              tunnel: [w645] -> w535
              tunnel: [w643] -> w534
              tunnel: [w641] -> w533
              tunnel: [w1406] -> w546
              tunnel: [w1407] -> w560
              tunnel: [w1408] -> w562
              tunnel: [w1409] -> w563
              tunnel: [w1410] -> w564
              tunnel: [w1411] -> w565
              tunnel: w538 -> [w1411]
              tunnel: w537 -> [w1410]
              tunnel: w536 -> [w1409]
              tunnel: w535 -> [w1408]
              tunnel: w534 -> [w1407]
              tunnel: w533 -> [w1406]
              tunnel: [w1405] -> w532
              tunnel: [w1404] -> w531
              tunnel: [w1403] -> w530
              tunnel: [w1402] -> w529
              tunnel: [w1401] -> w528
              tunnel: [w1400] -> w527
              frame #0 {
                n154 = local read "ScanMode"() -> (w573:i32)
                n155 = Equal?(x=w573, y=1) -> (x = y?=w572:bool)
                n156 = Equal?(x=w573, y=2) -> (x = y?=w571:bool)
                n157 = Unbundle(w577) -> (w576:dbl[][])
                n158 = Or(x=w572, y=w571) -> (x .or. y?=w570:bool)
                n159 = case shown="True" w570 {
                  tunnel: w585 -> [_ w599]
                  frame False {
                  }
                  frame True {
                    n160 = local read "YCoordCalBegin um"() -> (w617:dbl)
                    n161 = Index Array(array=w599, index (col) #1=0 ("index (row)"), index (col) #2=1 ("index (row)")) -> (element #1=w625:dbl[], element #2=w624:dbl[])  [unwired: 2 in]
                    n162 = local read "YCoordCalEnd um"() -> (w618:dbl)
                    n163 = Index Array(array=w625, index #1=0 ("index"), index #2=1 ("index")) -> (element #1=w623:dbl, element #2=w621:dbl)
                    n164 = Index Array(array=w624, index #1=0 ("index"), index #2=1 ("index")) -> (element #1=w622:dbl, element #2=w620:dbl)
                    n165 = local read "YStepSize um"() -> (w606:dbl)
                    n166 = local read "XStepSize um"() -> (w612:dbl)
                    n167 = Max & Min(x=w623, y=w622) -> (max(x,y)=w614:dbl, min(x,y)=w596:dbl)
                    n168 = Max & Min(x=w621, y=w620) -> (max(x,y)=w597:dbl, min(x,y)=w598:dbl)
                    n169 = Subtract(x=w618, y=w617) -> (x-y=w619:dbl)
                    n170 = Subtract(x=w614, y=w596) -> (x-y=w613:dbl)
                    n171 = Subtract(x=w619, y=w597) -> (x-y=w592:dbl)
                    n172 = Subtract(x=w597, y=w598) -> (x-y=w607:dbl)
                    n173 = Divide(x=w613, y=w612) -> (x/y=w616:dbl)
                    n174 = Divide(x=w607, y=w606) -> (x/y=w608:dbl)
                    n175 = Subtract(x=w596, y=1.0) -> (x-y=w595:dbl)
                    n176 = Subtract(x=w592, y=0.0) -> (x-y=w591:dbl)
                    n177 = Round To Nearest(number=w616) -> (nearest integer value=w615:dbl)
                    n178 = Round To Nearest(number=w608) -> (nearest integer value=w609:dbl)
                    n179 = local write "Adapted_XOffset um"(w595) -> ()
                    n180 = To Long Integer(number=w615) -> (32bit integer=w611:i32)
                    n181 = To Long Integer(number=w609) -> (32bit integer=w610:i32)
                    n182 = local write "Adapted_YOffset um"(w591) -> ()
                    n183 = local write "Adapted_XNum"(w611) -> ()
                    n184 = local write "Adapted_YNum"(w610) -> ()
                  }
                }
                n185 = Increment(x=w582) -> (x+1=w581:i32)
                n186 = Number To Decimal String(number=w584) -> (decimal integer string=w580:string)  [unwired: 1 in]
                n187 = Number To Decimal String(number=w581) -> (decimal integer string=w579:string)  [unwired: 1 in]
                n188 = Concatenate Strings(w579, " / " ("string"), w580) -> (w583:string)
                n189 = local write "RegionScanning"(w583) -> ()
              }
              frame #1 {
                n190 = local read "Adapted_XNum"() -> (w633:i32)
                n191 = local read "Adapted_YNum"() -> (w632:i32)
                n192 = local read "Retract (edge) um"() -> (w630:dbl)
                n193 = local read "Retract (flat) um"() -> (w631:dbl)
                n194 = call "HostDynamicRetractFormalization.vi"("Retract_Edge um"=w630, "Retract_Flat um"=w631, "YNum"=w632, "XNum"=w633, "InputLabel"=w629) -> ("OutputRetractMap um"=w628:dbl[][])  [unwired: 6 in]
                n195 = local write "Retract Map"(w628) -> ()
              }
              frame #2 {
                n196 = local read "FrameNum"() -> (w653:u32)
                n197 = for {
                  N: w653 -> [_]
                  tunnel: w652 -> [w687]
                  tunnel: w651 -> [w686]
                  tunnel: w650 -> [w685]
                  tunnel: w649 -> [w684]
                  tunnel: [w673] -> w648
                  tunnel: [w672] -> w647
                  tunnel: [w671] -> w646
                  tunnel: [w670] -> w645
                  tunnel: w644 -> [w667]
                  tunnel: [w664] -> w643
                  tunnel: w642 -> [w661]
                  tunnel: [w659] -> w641
                  tunnel: w640 -> [w658]
                  tunnel: w639 -> [w656]
                  i -> [w683]
                  stop <- w659 stop-if-true
                  n198 = flat-sequence {
                    tunnel: w683 -> [w706]
                    tunnel: w684 -> [w699]
                    tunnel: w685 -> [w701]
                    tunnel: w686 -> [w702]
                    tunnel: w687 -> [w703]
                    tunnel: [w700] -> w682
                    tunnel: [w698] -> w681
                    tunnel: [w697] -> w680
                    tunnel: [w699] -> w679
                    tunnel: [w706] -> w678
                    tunnel: w667 -> [w695]
                    tunnel: [w695] -> w666
                    tunnel: w661 -> [w693]
                    tunnel: [w693] -> w660
                    tunnel: w658 -> [w690]
                    tunnel: [w690] -> w657
                    tunnel: w656 -> [w689]
                    tunnel: [w689] -> w655
                    tunnel: [w752] -> w688
                    tunnel: w682 -> [w747]
                    tunnel: w681 -> [w746]
                    tunnel: w680 -> [w745]
                    tunnel: w679 -> [w744]
                    tunnel: w678 -> [w712]
                    tunnel: [w739] -> w677
                    tunnel: [w738] -> w676
                    tunnel: [w737] -> w675
                    tunnel: [w736] -> w674
                    tunnel: [w735] -> w669
                    tunnel: [w734] -> w668
                    tunnel: w666 -> [w724]
                    tunnel: [w723] -> w665
                    tunnel: [w719] -> w663
                    tunnel: [w718] -> w662
                    tunnel: w660 -> [w713]
                    tunnel: w657 -> [w711]
                    tunnel: w655 -> [w710]
                    tunnel: [w708] -> w654
                    tunnel: w688 -> [w1399]
                    tunnel: w677 -> [w1394]
                    tunnel: w676 -> [w1396]
                    tunnel: w675 -> [w1395]
                    tunnel: w674 -> [w1391]
                    tunnel: [w1394] -> w673
                    tunnel: [w1393] -> w672
                    tunnel: [w1392] -> w671
                    tunnel: [w1390] -> w670
                    tunnel: w669 -> [w1397]
                    tunnel: w668 -> [w1398]
                    tunnel: [w1398] -> w659
                    tunnel: w665 -> [w1388]
                    tunnel: [w1388] -> w664
                    tunnel: w663 -> [w1387]
                    tunnel: w662 -> [w1386]
                    tunnel: w654 -> [w1385]
                    frame #0 {
                      w691 = u8 2 ("Z Scale.Scale Fit")
                      w692 = TRUE ("Smooth Update")
                      w694 = FALSE ("Y Scale.Loose Fit")
                      n199 = local read "Adapted_YNum"() -> (w704:i32)
                      n200 = local read "Adapted_XNum"() -> (w705:i32)
                      n201 = property on="Pressure Slope Map" class="IntGraph (strict)"("XScale.Maximum"=w705, "YScale.Maximum"=w704, "YScale.LooseFit"=w694, "XScale.LooseFit"=w694, "ZScale.LooseFit"=w694, "Smooth Update"=w692, "ZScale.ScaleFit"=w691) -> ()  [unwired: 2 in, 2 out]
                      n202 = node(w703, w699, "db_start_frame_timer" ("function name"), w702, w701) -> (w700:refnum<k35>, w698:errorcluster, w697:refnum<k38>)  [unwired: 2 in, 2 out]
                      n203 = property on="Topography" class="IntGraph (strict)"("XScale.Maximum"=w705, "YScale.Maximum"=w704, "YScale.LooseFit"=w694, "XScale.LooseFit"=w694, "ZScale.LooseFit"=w694, "Smooth Update"=w692, "ZScale.ScaleFit"=w691) -> ()  [unwired: 2 in, 2 out]
                    }
                    frame #1 {
                      w716 = 100000.0
                      w717 = -100000.0
                      # "TTH param structure:\n0, 1: X, Y piezo voltage\n2, 3: X, Y piezo idx\n4: Z piezo probing voltage\n5: Z piezo final voltage\n6: baseline current\n7: circular buffer pointer idx\n(8-8107): Z voltage\n(8108-16207): current"
                      # "HTT param structure:\n0, 1: X, Y piezo voltage\n2, 3: X, Y piezo idx\n4: distance (piezo voltage) to the last point\n5: retract height, \nall negative cases won't trigger approach of z piezo\nif -20, keep z and move xy\nif -30, full retract for z and move xy"
                      n204 = local read "Adapted_XNum"() -> (w742:i32)
                      n205 = local read "Adapted_YNum"() -> (w741:i32)
                      n206 = Obtain Queue(name (unnamed)="data_array", element data type=dbl[] []) -> (queue out=w748:refnum<queue>)  [unwired: 3 in, 2 out]
                      n207 = New Data Value Reference(data value=FALSE) -> (data value reference=w749:refnum<data-value>)  [unwired: 1 in, 1 out]
                      n208 = Initialize Array(0.0, w742, w741) -> (w740:dbl[][])
                      n209 = flat-sequence {
                        tunnel: w749 -> [w1115]
                        tunnel: w748 -> [w1116]
                        tunnel: [w1116] -> w773
                        tunnel: [w1115] -> w771
                        tunnel: [w1114] -> w769
                        tunnel: [w1113] -> w766
                        tunnel: [w1108] -> w760
                        tunnel: [w1106] -> w759
                        tunnel: [w1101] -> w758
                        tunnel: [w1085] -> w757
                        tunnel: [w1098] -> w715
                        tunnel: [w1089] -> w714
                        tunnel: w713 -> [w1083]
                        tunnel: w712 -> [w1079]
                        tunnel: w711 -> [w1082]
                        tunnel: w710 -> [w1081]
                        tunnel: [w1074] -> w709
                        tunnel: [w1060] -> w707
                        tunnel: [w1171] -> w775
                        tunnel: [w1170] -> w774
                        tunnel: w773 -> [w1169]
                        tunnel: [w1169] -> w772
                        tunnel: w771 -> [w1162]
                        tunnel: [w1162] -> w770
                        tunnel: w769 -> [w1152]
                        tunnel: [w1164] -> w768
                        tunnel: [w1163] -> w767
                        tunnel: w766 -> [w1161]
                        tunnel: [w1161] -> w765
                        tunnel: [w1162] -> w764
                        tunnel: [w1160] -> w763
                        tunnel: [0] -> w762
                        tunnel: [w1158] -> w761
                        tunnel: w760 -> [w1157]
                        tunnel: w759 -> [w1156]
                        tunnel: w758 -> [w1155]
                        tunnel: w757 -> [w1153]
                        tunnel: [0] -> w751
                        tunnel: [w1153] -> w750
                        tunnel: w715 -> [w1151]
                        tunnel: w714 -> [w1150]
                        tunnel: w709 -> [_]
                        tunnel: w707 -> [w1148]
                        tunnel: w775 -> [w1197]
                        tunnel: w774 -> [w1196]
                        tunnel: w772 -> [w1195]
                        tunnel: w770 -> [w1194]
                        tunnel: w768 -> [w1193]
                        tunnel: w767 -> [w1192]
                        tunnel: w765 -> [w1191]
                        tunnel: w764 -> [w1190]
                        tunnel: w763 -> [w1189]
                        tunnel: w762 -> [w1188]
                        tunnel: w761 -> [w1187]
                        tunnel: [w1186] -> w756
                        tunnel: [w1185] -> w755
                        tunnel: [w1184] -> w754
                        tunnel: [w1183] -> w753
                        tunnel: w751 -> [w1182]
                        tunnel: w750 -> [w1181]
                        tunnel: [w1180] -> w733
                        tunnel: [w1179] -> w722
                        tunnel: [w1363] -> w732
                        tunnel: [w1362] -> w730
                        tunnel: [w1361] -> w728
                        tunnel: [w1359] -> w726
                        tunnel: w733 -> [w1358]
                        tunnel: w753 -> [w1360]
                        tunnel: w754 -> [w1361]
                        tunnel: w755 -> [w1362]
                        tunnel: w756 -> [w1363]
                        tunnel: w722 -> [w1357]
                        tunnel: [w1357] -> w720
                        tunnel: w732 -> [w1377]
                        tunnel: [w1377] -> w731
                        tunnel: w730 -> [w1376]
                        tunnel: [w1376] -> w729
                        tunnel: w728 -> [w1375]
                        tunnel: [w1375] -> w727
                        tunnel: w726 -> [w1374]
                        tunnel: [w1374] -> w725
                        tunnel: [w1372] -> w721
                        tunnel: w720 -> [w1372]
                        tunnel: w731 -> [w1379]
                        tunnel: w729 -> [w1378]
                        tunnel: w727 -> [w1383]
                        tunnel: w725 -> [w1382]
                        tunnel: [w1382] -> w752
                        tunnel: [w1381] -> w735
                        tunnel: w721 -> [w1380]
                        tunnel: [w1380] -> w719
                        frame #0 {
                          n210 = local read "ScanMode"() -> (w1084:i32)
                          n211 = local read "FrameNum"() -> (w1078:u32)
                          n212 = Equal?(x=w1084, y=3) -> (x = y?=w1067:bool)
                          n213 = Decrement(x=w1078) -> (x-1=w1077:u32)
                          n214 = Decrement(x=w1081) -> (x-1=w1080:i32)
                          n215 = local read "Adapted_XNum"() -> (w1100:i32)
                          n216 = local read "Adapted_YNum"() -> (w1099:i32)
                          n217 = Equal?(x=w1082, y=w1080) -> (x = y?=w1075:bool)
                          n218 = case shown="3" w1084 {
                            tunnel: [w1117 w1126 w1134 w1145] -> w1113
                            tunnel: w1083 -> [_ _ _ _]
                            frame 0, Default {
                              n219 = local read "Adapted_XNum"() -> (w1124:i32)
                              n220 = local read "Adapted_YNum"() -> (w1123:i32)
                              n221 = local read "Adapted_YOffset um"() -> (w1120:dbl)
                              n222 = local read "Adapted_XOffset um"() -> (w1119:dbl)
                              n223 = local read "Retract (flat) um"() -> (w1118:dbl)
                              n224 = local read "XStepSize um"() -> (w1122:dbl)
                              n225 = local read "YStepSize um"() -> (w1121:dbl)
                              n226 = call "xy_raster_scan.vi"("Retract um"=w1118, "YOffset um"=w1120, "XOffset um"=w1119, "YStepSize um"=w1121, "XStepSize um"=w1122, "YNum"=w1123, "XNum"=w1124) -> ("Converted_HTT_Params"=w1117:fxp<+/-,48,16>[])  [unwired: 4 in]
                            }
                            frame 1 {
                              n227 = local read "Adapted_XOffset um"() -> (w1130:dbl)
                              n228 = local read "Adapted_YOffset um"() -> (w1127:dbl)
                              n229 = local read "Retract (edge) um"() -> (w1125:dbl)
                              n230 = local read "Adapted_XNum"() -> (w1132:i32)
                              n231 = local read "Adapted_YNum"() -> (w1131:i32)
                              n232 = local read "XStepSize um"() -> (w1129:dbl)
                              n233 = local read "YStepSize um"() -> (w1128:dbl)
                              n234 = call "xy_raster_scan.vi"("Retract um"=w1125, "YOffset um"=w1127, "XOffset um"=w1130, "YStepSize um"=w1128, "XStepSize um"=w1129, "YNum"=w1131, "XNum"=w1132) -> ("Converted_HTT_Params"=w1126:fxp<+/-,48,16>[])  [unwired: 4 in]
                            }
                            frame 2 {
                              n235 = local read "Adapted_XOffset um"() -> (w1138:dbl)
                              n236 = local read "Adapted_YOffset um"() -> (w1135:dbl)
                              n237 = local read "Retract (edge) um"() -> (w1133:dbl)
                              n238 = local read "Adapted_XNum"() -> (w1140:i32)
                              n239 = local read "Adapted_YNum"() -> (w1139:i32)
                              n240 = local read "XStepSize um"() -> (w1137:dbl)
                              n241 = local read "YStepSize um"() -> (w1136:dbl)
                              n242 = call "xy_raster_scan.vi"("Retract um"=w1133, "YOffset um"=w1135, "XOffset um"=w1138, "YStepSize um"=w1136, "XStepSize um"=w1137, "YNum"=w1139, "XNum"=w1140) -> ("Converted_HTT_Params"=w1134:fxp<+/-,48,16>[])  [unwired: 4 in]
                            }
                            frame 3 {
                              w1144 = 0.0 ("XStepSize um")
                              w1141 = 1 ("YNum")
                              w1142 = 400 ("XNum")
                              n243 = local read "XOffset um"() -> (w1146:dbl)
                              n244 = local read "YOffset um"() -> (w1147:dbl)
                              n245 = local write "Adapted_XNum"(w1142) -> ()
                              n246 = local write "Adapted_YNum"(w1141) -> ()
                              n247 = call "xy_raster_scan.vi"("Retract um"=2.0, "YOffset um"=w1147, "XOffset um"=w1146, "YStepSize um"=w1144, "XStepSize um"=w1144, "YNum"=w1141, "XNum"=w1142) -> ("Converted_HTT_Params"=w1145:fxp<+/-,48,16>[])  [unwired: 4 in]
                            }
                          }
                          n248 = Equal?(x=w1079, y=w1077) -> (x = y?=w1076:bool)
                          n249 = Multiply(x=w1100, y=w1099) -> (x*y=w1087:i32)
                          n250 = local read "NF_AppRate um/s"() -> (w1070:dbl)
                          n251 = local read "FF_AppRate um/s"() -> (w1066:dbl)
                          n252 = local read "RetRate um/s"() -> (w1073:dbl)
                          n253 = local read "NF_Threshold %"() -> (w1093:dbl)
                          n254 = local read "FF_Threshold %"() -> (w1097:dbl)
                          n255 = Select(t=400, s=w1067, f=w1087) -> (s? t:f=w1085:i32)
                          n256 = And(x=w1076, y=w1075) -> (x .and. y?=w1074:bool)
                          n257 = Divide(x=25.0, y=0.032768) -> (x/y=w1102:dbl)
                          n258 = local read "Turning Distance um"() -> (w1063:dbl)
                          n259 = Select(t=15.0, s=w1067, f=w1073) -> (s? t:f=w1071:dbl)
                          n260 = Select(t=3.0, s=w1067, f=w1070) -> (s? t:f=w1068:dbl)
                          n261 = Select(t=5.0, s=w1067, f=w1066) -> (s? t:f=w1064:dbl)
                          n262 = Divide(x=w1097, y=100.0) -> (x/y=w1096:dbl)
                          n263 = Divide(x=w1093, y=100.0) -> (x/y=w1092:dbl)
                          n264 = Divide(x=w1102, y=w1064) -> (x/y=w1110:dbl)
                          n265 = Divide(x=w1102, y=w1068) -> (x/y=w1103:dbl)
                          n266 = Divide(x=w1102, y=w1071) -> (x/y=w1105:dbl)
                          n267 = Select(t=2, s=w1067, f=1) -> (s? t:f=w1089:i32)
                          n268 = Divide(x=w1063, y=2.5) -> (x/y=w1061:dbl)
                          n269 = Round To Nearest(number=w1110) -> (nearest integer value=w1109:dbl)
                          n270 = To Fixed-Point(number=w1096) -> (fixed-point=w1114:fxp<+/-,48,16>)  [unwired: 1 in]
                          n271 = To Fixed-Point(number=w1092) -> (fixed-point=w1098:fxp<+/-,48,16>)  [unwired: 1 in]
                          n272 = Round To Nearest(number=w1103) -> (nearest integer value=w1107:dbl)
                          n273 = Round To Nearest(number=w1105) -> (nearest integer value=w1104:dbl)
                          n274 = To Long Integer(number=w1107) -> (32bit integer=w1106:i32)
                          n275 = To Long Integer(number=w1104) -> (32bit integer=w1101:i32)
                          n276 = To Long Integer(number=w1109) -> (32bit integer=w1108:i32)
                          n277 = To Fixed-Point(number=w1061) -> (fixed-point=w1060:fxp<+/-,48,16>)  [unwired: 1 in]
                        }
                        frame #1 {
                          w1149 = TRUE ("InitScan")
                          n278 = xnode "Open FPGA VI Reference"("resource name"=tag "RIO0") -> ("FPGA VI Reference Out"=w1168:refnum<k20>, "error out"=w1167:errorcluster)  [unwired: 1 in]
                          n279 = xnode "Read/Write Control"("FPGA VI Reference In"=w1168, "error in"=w1167, "Recording Threshold"=w1152, "Halting Threshold"=w1151, "AppRate_FF us"=w1157, "AppRate_NF us"=w1156, "RetRate us"=w1155, "TotalPoints"=w1153, "DelayPoints"=w1150, "InitScan"=w1149, "LastScan"=w1149, "Turning Distance"=w1148) -> ("FPGA VI Reference Out"=w1177:refnum<k20>, "error out"=w1176:errorcluster)
                          n280 = xnode "Invoke Method"("FPGA VI Reference In"=w1168, "error in"=w1167, "Data"=fxp<+/-,48,16>[] [], "Timeout (ms)"=0) -> ("FPGA VI Reference Out"=w1164:refnum<k20>, "error out"=w1163:errorcluster, "Empty Elements Remaining"=w1158:u32)
                          n281 = Scale By Power Of 2(n=u32 18 ("Requested Depth"), x=u32 1 ("Requested Depth")) -> (x*2^n=w1173:u32)
                          n282 = xnode "Invoke Method"("FPGA VI Reference In"=w1177, "error in"=w1176, "Requested Depth"=w1173) -> ("FPGA VI Reference Out"=w1171:refnum<k20>, "error out"=w1170:errorcluster, "Actual Depth"=→"FPGA_Host_Buf_Depth":u32)
                          n283 = Array Size(array=w1161) -> (size(s)=w1160:i32)
                        }
                        frame #2 {
                          n284 = while {
                            tunnel: w1193 -> [w1215]
                            tunnel: w1192 -> [w1214]
                            tunnel: w1191 -> [w1211]
                            tunnel: w1190 -> [w1210]
                            tunnel: w1189 -> [w1209]
                            shift-right: [w1202] -> _
                            shift-left: w1188 -> [w1208]
                            tunnel: w1187 -> [w1207]
                            stop <- w1198 stop-if-true
                            n285 = flat-sequence {
                              tunnel: w1215 -> [w1239]
                              tunnel: w1214 -> [w1238]
                              tunnel: [w1233] -> w1213
                              tunnel: [w1232] -> w1212
                              tunnel: w1211 -> [w1221]
                              tunnel: w1210 -> [w1231]
                              tunnel: w1209 -> [w1230]
                              tunnel: w1208 -> [w1225]
                              tunnel: w1207 -> [w1229]
                              tunnel: [w1225] -> w1206
                              tunnel: [w1222] -> w1205
                              tunnel: [w1221] -> w1204
                              tunnel: [w1217] -> w1201
                              tunnel: [w1216] -> w1200
                              tunnel: w1213 -> [w1248]
                              tunnel: w1212 -> [w1247]
                              tunnel: w1206 -> [w1246]
                              tunnel: w1205 -> [w1245]
                              tunnel: w1204 -> [w1244]
                              tunnel: [w1243] -> w1203
                              tunnel: w1201 -> [w1242]
                              tunnel: w1200 -> [w1241]
                              tunnel: [w1241] -> w1199
                              tunnel: w1203 -> [w1259]
                              tunnel: [w1259] -> w1202
                              tunnel: w1199 -> [w1258]
                              tunnel: [w1258] -> w1198
                              frame #0 {
                                w1223 = u32 128 ("y")
                                n286 = in-place {
                                in-place-border: [w1240] -> w1219
                                n287 = in-place-dvr #1(w1231) -> (w1240:bool)  [unwired: 1 out]
                                n288 = in-place-dvr #1(w1240) -> ()  [unwired: 2 out]
                                }
                                n289 = xnode "Invoke Method"("FPGA VI Reference In"=w1239, "error in"=w1238, "Data"=fxp<+/-,48,16>[] [], "Timeout (ms)"=0) -> ("FPGA VI Reference Out"=w1235:refnum<k20>, "error out"=w1234:errorcluster, "Empty Elements Remaining"=w1228:u32)
                                n290 = Subtract(x=w1230, y=w1225) -> (x-y=w1224:u32)
                                n291 = Subtract(x=w1229, y=w1228) -> (x-y=w1227:u32)
                                n292 = Less Or Equal?(x=w1227, y=w1223) -> (x <= y?=w1226:bool)
                                n293 = Less Or Equal?(x=w1224, y=w1223) -> (x <= y?=w1218:bool)
                                n294 = Or(x=w1226, y=w1218) -> (x .or. y?=w1217:bool)
                                n295 = xnode "Read/Write Control"("FPGA VI Reference In"=w1235, "error in"=w1234) -> ("FPGA VI Reference Out"=w1233:refnum<k20>, "error out"=w1232:errorcluster, "TargetDone?"=w1220:bool)
                                n296 = Select(t=w1224, s=w1218, f=w1223) -> (s? t:f=w1222:u32)
                                n297 = Compound Arithmetic op=OR(w1220, w1218, w1219) -> (w1216:bool)
                              }
                              frame #1 {
                                n298 = case shown="True" w1242 {
                                tunnel: w1248 -> [_ w1257]
                                tunnel: w1247 -> [_ w1256]
                                tunnel: w1246 -> [w1249 w1252]
                                tunnel: w1245 -> [_ w1251]
                                tunnel: w1244 -> [_ w1253]
                                tunnel: [w1249 w1254] -> w1243
                                frame False {
                                }
                                frame True {
                                n299 = Array Subset(array=w1253, index=w1252, length=w1251) -> (w1250:fxp<+/-,48,16>[])
                                n300 = Add(x=w1251, y=w1252) -> (x+y=w1254:u32)
                                "HTT_Buffer_Write" <- w1254
                                n301 = xnode "Invoke Method"("FPGA VI Reference In"=w1257, "error in"=w1256, "Data"=w1250, "Timeout (ms)"=10000) -> ()  [unwired: 3 out]
                                }
                                }
                              }
                              frame #2 {
                                n302 = Wait (ms)(milliseconds to wait=u32 100) -> ()  [unwired: 1 out]
                              }
                            }
                          }
                          n303 = while {
                            tunnel: w1197 -> [w1290]
                            tunnel: w1196 -> [w1289]
                            tunnel: w1195 -> [w1286]
                            tunnel: w1194 -> [w1285]
                            tunnel: [w1278] -> w1186
                            tunnel: [w1277] -> w1185
                            tunnel: [w1275] -> w1184
                            tunnel: [w1273] -> w1183
                            shift-right: [w1269] -> _
                            shift-left: w1182 -> [w1272]
                            tunnel: w1181 -> [w1265]
                            tunnel: [w1262] -> w1180
                            tunnel: [w1261] -> w1179
                            stop <- w1266 stop-if-true
                            n304 = flat-sequence {
                              tunnel: w1290 -> [w1309]
                              tunnel: w1289 -> [w1308]
                              tunnel: [w1303] -> w1288
                              tunnel: [w1302] -> w1287
                              tunnel: w1286 -> [w1298]
                              tunnel: w1285 -> [w1296]
                              tunnel: [w1298] -> w1284
                              tunnel: [w1297] -> w1283
                              tunnel: [w1295] -> w1282
                              tunnel: [w1294] -> w1279
                              tunnel: w1272 -> [w1293]
                              tunnel: [w1293] -> w1271
                              tunnel: [w1291] -> w1268
                              tunnel: w1265 -> [w1292]
                              tunnel: [w1292] -> w1264
                              tunnel: w1288 -> [w1323]
                              tunnel: w1287 -> [w1322]
                              tunnel: w1284 -> [w1321]
                              tunnel: w1283 -> [w1320]
                              tunnel: w1282 -> [w1319]
                              tunnel: [w1318] -> w1281
                              tunnel: [w1317] -> w1280
                              tunnel: w1279 -> [w1316]
                              tunnel: [w1316] -> w1276
                              tunnel: [w1315] -> w1274
                              tunnel: w1271 -> [w1314]
                              tunnel: [w1313] -> w1270
                              tunnel: w1268 -> [w1312]
                              tunnel: [w1312] -> w1267
                              tunnel: w1264 -> [w1311]
                              tunnel: [w1311] -> w1263
                              tunnel: w1281 -> [w1355]
                              tunnel: w1280 -> [w1354]
                              tunnel: [w1355] -> w1278
                              tunnel: [w1354] -> w1277
                              tunnel: [w1353] -> w1275
                              tunnel: w1276 -> [w1353]
                              tunnel: w1274 -> [w1352]
                              tunnel: [w1352] -> w1273
                              tunnel: w1270 -> [w1350]
                              tunnel: [w1350] -> w1269
                              tunnel: w1267 -> [w1348]
                              tunnel: [w1351] -> w1266
                              tunnel: w1263 -> [w1349]
                              tunnel: [w1348] -> w1262
                              tunnel: [w1347] -> w1261
                              frame #0 {
                                w1301 = 16384
                                w1305 = u32 0 ("Number of Elements")
                                n305 = in-place {
                                in-place-border: [w1310] -> w1291
                                n306 = in-place-dvr #2(w1296) -> (w1310:bool)  [unwired: 1 out]
                                n307 = in-place-dvr #2(w1310) -> (w1294:refnum<data-value>)  [unwired: 1 out]
                                }
                                n308 = xnode "Read/Write Control"("FPGA VI Reference In"=w1309, "error in"=w1308, "stop"=w1291) -> ("FPGA VI Reference Out"=w1307:refnum<k20>, "error out"=w1306:errorcluster)
                                n309 = xnode "Invoke Method"("FPGA VI Reference In"=w1307, "error in"=w1306, "Number of Elements"=w1305, "Timeout (ms)"=w1305) -> ("FPGA VI Reference Out"=w1303:refnum<k20>, "error out"=w1302:errorcluster, "Elements Remaining"=w1304:u32)  [unwired: 1 out]
                                n310 = Quotient & Remainder(x=w1304, y=w1301) -> (floor(x/y)=w1300:u32)  [unwired: 1 out]
                                n311 = Multiply(x=w1301, y=w1300) -> (x*y=w1295:u32)
                                n312 = Greater Than 0?(x=w1300) -> (x > 0?=w1299:bool)
                                n313 = Compound Arithmetic op=AND(w1299, invert w1291) -> (w1297:bool)
                              }
                              frame #1 {
                                n314 = case shown="True" w1320 {
                                tunnel: w1323 -> [w1327 w1343]
                                tunnel: w1322 -> [w1326 w1342]
                                tunnel: w1321 -> [w1325 w1336]
                                tunnel: w1319 -> [_ w1338]
                                tunnel: [w1327 w1340] -> w1318
                                tunnel: [w1326 w1339] -> w1317
                                tunnel: [w1325 w1331] -> w1315
                                tunnel: w1314 -> [w1324 w1330]
                                tunnel: [w1324 w1328] -> w1313
                                frame False {
                                }
                                frame True {
                                w1333 = 16384
                                n315 = xnode "Invoke Method"("FPGA VI Reference In"=w1343, "error in"=w1342, "Number of Elements"=w1338, "Timeout (ms)"=10000) -> ("FPGA VI Reference Out"=w1340:refnum<k20>, "error out"=w1339:errorcluster, "Data"=w1337:fxp<+/-,48,16>[])  [unwired: 1 out]
                                n316 = To Double Precision Float(number=w1337) -> (double precision float=w1334:dbl[])
                                n317 = Array Size(array=w1334) -> (size(s)=w1335:i32)
                                n318 = Quotient & Remainder(x=w1335, y=w1333) -> (floor(x/y)=w1329:i32)  [unwired: 1 out]
                                n319 = Add(x=w1330, y=w1329) -> (x+y=w1328:i32)
                                n320 = Reshape Array(w1334, w1329, w1333) -> (w1332:dbl[][])
                                n321 = for {
                                N: w1329 -> [_]
                                tunnel: w1336 -> [w1346]
                                tunnel: w1332 -> [w1345] mode=indexing
                                tunnel: [w1344] -> w1331
                                n322 = Enqueue Element(queue=w1346, element=w1345) -> (queue out=w1344:refnum<queue>)  [unwired: 2 in, 2 out]
                                }
                                }
                                }
                              }
                              frame #2 {
                                n323 = Greater Or Equal?(x=w1350, y=w1349) -> (x >= y?=w1347:bool)
                                n324 = Wait (ms)(milliseconds to wait=u32 20) -> ()  [unwired: 1 out]
                                n325 = Or(x=w1347, y=w1348) -> (x .or. y?=w1351:bool)
                                "Scanned Points" <- w1350
                              }
                            }
                          }
                        }
                        frame #3 {
                          n326 = case shown="False" w1358 {
                            tunnel: w1360 -> [w1365 w1371]
                            tunnel: [w1364 w1371] -> w1359
                            frame False {
                              n327 = while {
                                tunnel: w1365 -> [w1370]
                                tunnel: [w1369] -> w1364
                                stop <- w1367 stop-if-true
                                n328 = Get Queue Status(queue=w1370) -> (queue out=w1369:refnum<queue>, # elements in queue=w1368:i32)  [unwired: 2 in, 6 out]
                                n329 = Less Or Equal To 0?(x=w1368) -> (x <= 0?=w1367:bool)
                                n330 = Wait (ms)(milliseconds to wait=u32 100) -> ()  [unwired: 1 out]
                              }
                            }
                            frame True {
                            }
                          }
                        }
                        frame #4 {
                          n331 = Wait (ms)(milliseconds to wait=u32 500) -> ()  [unwired: 1 out]
                        }
                        frame #5 {
                          n332 = in-place {
                            n333 = in-place-dvr #3(w1383) -> ()  [unwired: 2 out]
                            n334 = in-place-dvr #3(TRUE ("data value")) -> (w1381:refnum<data-value>)  [unwired: 1 out]
                          }
                          n335 = xnode "Close FPGA VI Reference"("FPGA VI Reference In"=w1379, "error in"=w1378) -> ()  [unwired: 1 out]
                        }
                      }
                      n336 = flat-sequence {
                        tunnel: w749 -> [w801]
                        tunnel: w748 -> [w800]
                        tunnel: w747 -> [w799]
                        tunnel: w746 -> [w798]
                        tunnel: w745 -> [w797]
                        tunnel: w744 -> [w796]
                        tunnel: [w795] -> w739
                        tunnel: [w794] -> w738
                        tunnel: [w793] -> w737
                        tunnel: [w792] -> w736
                        tunnel: w712 -> [w791]
                        tunnel: w740 -> [w790]
                        tunnel: w740 -> [w789]
                        tunnel: w717 -> [w788]
                        tunnel: w716 -> [w787]
                        tunnel: w717 -> [w786]
                        tunnel: w716 -> [w785]
                        tunnel: [w784] -> w734
                        tunnel: w724 -> [w783]
                        tunnel: [w782] -> w723
                        tunnel: [w781] -> w718
                        tunnel: w711 -> [w780]
                        tunnel: [w779] -> w708
                        frame #0 {
                          n337 = while {
                            tunnel: w801 -> [w864]
                            tunnel: w800 -> [w863]
                            tunnel: w799 -> [w862]
                            tunnel: w798 -> [w861]
                            tunnel: w797 -> [w860]
                            tunnel: w796 -> [w856]
                            tunnel: [w850] -> w795
                            tunnel: [w849] -> w794
                            tunnel: [w848] -> w793
                            tunnel: [w847] -> w792
                            tunnel: w791 -> [w843]
                            shift-right: [w833] -> _
                            shift-left: w790 -> [w841]
                            shift-right: [w831] -> _
                            shift-left: w789 -> [w836]
                            shift-right: [w821] -> _
                            shift-left: w788 -> [w830]
                            shift-right: [w819] -> _
                            shift-left: w787 -> [w829]
                            shift-right: [w817] -> _
                            shift-left: w786 -> [w826]
                            shift-right: [w815] -> _
                            shift-left: w785 -> [w825]
                            tunnel: [w812] -> w784
                            tunnel: w783 -> [w811]
                            tunnel: [w808] -> w782
                            tunnel: [w806] -> w781
                            tunnel: w780 -> [w805]
                            tunnel: [w802] -> w779
                            stop <- w838 stop-if-true
                            n338 = flat-sequence {
                              tunnel: w864 -> [w887]
                              tunnel: w863 -> [w882]
                              tunnel: w862 -> [w886]
                              tunnel: w861 -> [w885]
                              tunnel: w860 -> [w884]
                              tunnel: [w886] -> w859
                              tunnel: [w885] -> w858
                              tunnel: [w884] -> w857
                              tunnel: w856 -> [w883]
                              tunnel: [w883] -> w855
                              tunnel: [w881] -> w846
                              tunnel: [w880] -> w845
                              tunnel: [w879] -> w844
                              tunnel: w843 -> [w878]
                              tunnel: [w878] -> w842
                              tunnel: w841 -> [w876]
                              tunnel: [w877] -> w840
                              tunnel: [w876] -> w837
                              tunnel: w836 -> [w875]
                              tunnel: [w875] -> w835
                              tunnel: w830 -> [w874]
                              tunnel: w829 -> [w873]
                              tunnel: [w874] -> w828
                              tunnel: [w873] -> w827
                              tunnel: w826 -> [w872]
                              tunnel: w825 -> [w871]
                              tunnel: [w872] -> w824
                              tunnel: [w871] -> w823
                              tunnel: [w870] -> w814
                              tunnel: w811 -> [w869]
                              tunnel: [w866] -> w810
                              tunnel: w805 -> [w865]
                              tunnel: [w865] -> w804
                              tunnel: w859 -> [w920]
                              tunnel: w858 -> [w919]
                              tunnel: w857 -> [w918]
                              tunnel: w855 -> [w917]
                              tunnel: [w916] -> w854
                              tunnel: [w915] -> w853
                              tunnel: [w914] -> w852
                              tunnel: [w913] -> w851
                              tunnel: w846 -> [w912]
                              tunnel: w845 -> [w911]
                              tunnel: w844 -> [w910]
                              tunnel: w842 -> [w909]
                              tunnel: w840 -> [w908]
                              tunnel: [w908] -> w839
                              tunnel: w837 -> [w907]
                              tunnel: w835 -> [w906]
                              tunnel: [w905] -> w834
                              tunnel: [w904] -> w832
                              tunnel: w828 -> [w903]
                              tunnel: w827 -> [w902]
                              tunnel: w824 -> [w901]
                              tunnel: w823 -> [w900]
                              tunnel: [w899] -> w822
                              tunnel: [w898] -> w820
                              tunnel: [w897] -> w818
                              tunnel: [w896] -> w816
                              tunnel: w814 -> [w895]
                              tunnel: [w895] -> w813
                              tunnel: w810 -> [w894]
                              tunnel: [w894] -> w809
                              tunnel: [w893] -> w807
                              tunnel: w804 -> [w892]
                              tunnel: [w891] -> w803
                              tunnel: w854 -> [w1057]
                              tunnel: w853 -> [w1056]
                              tunnel: w852 -> [w1055]
                              tunnel: w851 -> [w1058]
                              tunnel: [w1058] -> w850
                              tunnel: [w1057] -> w849
                              tunnel: [w1056] -> w848
                              tunnel: [w1055] -> w847
                              tunnel: [w1054] -> w838
                              tunnel: w839 -> [w1054]
                              tunnel: w834 -> [w1053]
                              tunnel: [w1053] -> w833
                              tunnel: w832 -> [w1052]
                              tunnel: [w1052] -> w831
                              tunnel: w822 -> [w1051]
                              tunnel: [w1051] -> w821
                              tunnel: w820 -> [w1050]
                              tunnel: [w1050] -> w819
                              tunnel: w818 -> [w1049]
                              tunnel: [w1049] -> w817
                              tunnel: w816 -> [w1048]
                              tunnel: [w1048] -> w815
                              tunnel: w813 -> [w1047]
                              tunnel: [w1047] -> w812
                              tunnel: w809 -> [w1046]
                              tunnel: [w1046] -> w808
                              tunnel: w807 -> [w1045]
                              tunnel: [w1045] -> w806
                              tunnel: w803 -> [w1044]
                              tunnel: [w1044] -> w802
                              frame #0 {
                                # "topography max min"
                                # "pressure slope map"
                                # "topography"
                                n339 = Get Queue Status(queue=w869) -> (queue out=w866:refnum<queue>, # elements in queue=w868:i32)  [unwired: 2 in, 6 out]
                                n340 = Greater Than 0?(x=w868) -> (x > 0?=w867:bool)
                                n341 = Get Queue Status(queue=w882) -> (queue out=w880:refnum<queue>, # elements in queue=w879:i32)  [unwired: 2 in, 6 out]
                                n342 = in-place {
                                in-place-border: w867 -> [w888]
                                in-place-border: [w889] -> w877
                                in-place-border: [w888] -> w870
                                n343 = in-place-dvr #4(w887) -> (w890:bool)  [unwired: 1 out]
                                n344 = Or(x=w890, y=w888) -> (x .or. y?=w889:bool)
                                n345 = in-place-dvr #4(w889) -> ()  [unwired: 2 out]
                                }
                                n346 = Greater Than 0?(x=w879) -> (x > 0?=w881:bool)
                              }
                              frame #1 {
                                n347 = case shown="True" w912 {
                                tunnel: w920 -> [w931 w961]
                                tunnel: w919 -> [w930 w960]
                                tunnel: w918 -> [w929 w959]
                                tunnel: w917 -> [w932 w955]
                                tunnel: [w931 w958] -> w916
                                tunnel: [w930 w957] -> w915
                                tunnel: [w929 w956] -> w914
                                tunnel: [w932 w954] -> w913
                                tunnel: w911 -> [_ w952]
                                tunnel: w910 -> [_ w953]
                                tunnel: w909 -> [w922 w951]
                                tunnel: w907 -> [w928 w950]
                                tunnel: w906 -> [w927 w949]
                                tunnel: [w928 w936] -> w905
                                tunnel: [w927 w935] -> w904
                                tunnel: w903 -> [w926 w945]
                                tunnel: w902 -> [w925 w944]
                                tunnel: w901 -> [w924 w943]
                                tunnel: w900 -> [w923 w942]
                                tunnel: [w926 w941] -> w899
                                tunnel: [w925 w940] -> w898
                                tunnel: [w924 w939] -> w897
                                tunnel: [w923 w938] -> w896
                                tunnel: [w922 w937] -> w893
                                tunnel: w892 -> [w921 w934]
                                tunnel: [w921 w933] -> w891
                                frame False {
                                }
                                frame True {
                                n348 = for {
                                N: w953 -> [_]
                                tunnel: w955 -> [w1029]
                                tunnel: [w1029] -> w954
                                tunnel: w961 -> [w1036]
                                tunnel: [w1032] -> w958
                                tunnel: w960 -> [w1034]
                                tunnel: [w1031] -> w957
                                tunnel: w959 -> [w1033]
                                tunnel: [w1030] -> w956
                                tunnel: w952 -> [w1028]
                                tunnel: w951 -> [w976]
                                shift-right: [w995] -> w936
                                shift-left: w950 -> [w996]
                                shift-right: [w993] -> w935
                                shift-left: w949 -> [w994]
                                tunnel: [w972] -> w948
                                tunnel: [w973] -> w947
                                shift-right: [w991] -> w941
                                shift-left: w945 -> [w992]
                                shift-right: [w989] -> w940
                                shift-left: w944 -> [w990]
                                shift-right: [w985] -> w939
                                shift-left: w943 -> [w988]
                                shift-right: [w984] -> w938
                                shift-left: w942 -> [w987]
                                tunnel: [w983] -> w937
                                tunnel: w934 -> [w975]
                                tunnel: [w975] -> w933
                                w998 = T3 0 items=["Least Square", "Least Absolute Residual", "Bisquare"] ("method")
                                n349 = Dequeue Element(queue=w1028) -> (element=w1019:dbl[])  [unwired: 2 in, 3 out]
                                n350 = Array Subset(array=w1019, index=8, length=8100 ("index")) -> (w1012:dbl[])
                                n351 = Array Subset(array=w1019, index=8108, length=8100 ("index")) -> (w1013:dbl[])
                                n352 = Index Array(array=w1019, index #1=0 ("index"), index #2=1 ("index"), index #3=2 ("index"), index #4=3 ("index"), index #5=4 ("index"), index #6=5 ("index"), index #7=6 ("index"), index #8=7 ("index")) -> (element #1=w1010:dbl, element #2=w1008:dbl, element #3=w1007:dbl, element #4=w1005:dbl, element #5=w963:dbl, element #6=w967:dbl, element #7=w968:dbl, element #8=w969:dbl)
                                n353 = To Long Integer(number=w969) -> (32bit integer=w971:i32)
                                n354 = Search 1D Array(1D array=w1012, element=-100.0) -> (index of element=w1011:i32)  [unwired: 1 in]
                                n355 = Equal?(x=w1011, y=-1) -> (x = y?=w1014:bool)
                                n356 = To Long Integer(number=w1007) -> (32bit integer=w979:i32)
                                n357 = To Long Integer(number=w1005) -> (32bit integer=w980:i32)
                                n358 = case shown="False" w1014 {
                                tunnel: w1013 -> [w1040 w1042]
                                tunnel: w1012 -> [w1041 w1043]
                                tunnel: w1011 -> [w1037 _]
                                tunnel: [w1039 w1043] -> w999
                                tunnel: [w1038 w1042] -> w973
                                frame False {
                                n359 = Split 1D Array(array=w1041, index=w1037) -> (first subarray=w1039:dbl[])  [unwired: 1 out]
                                n360 = Split 1D Array(array=w1040, index=w1037) -> (first subarray=w1038:dbl[])  [unwired: 1 out]
                                }
                                frame True {
                                }
                                }
                                n361 = Multiply(x=w1010, y=10.0) -> (x*y=w977:dbl)
                                n362 = Multiply(x=w963, y=2.5) -> (x*y=w965:dbl)
                                n363 = Multiply(x=w1008, y=10.0) -> (x*y=w978:dbl)
                                n364 = Multiply(x=w967, y=2.5) -> (x*y=w1003:dbl)
                                n365 = Subtract(x=25.0, y=w965) -> (x-y=w962:dbl)
                                n366 = Subtract(x=25.0, y=w1003) -> (x-y=w970:dbl)
                                n367 = Multiply(x=w999, y=2.5) -> (x*y=w997:dbl[])
                                n368 = Array Size(array=w973) -> (size(s)=→"Signal Size":i32)
                                n369 = Subtract(x=25.0, y=w997) -> (x-y=w972:dbl[])
                                n370 = call <vilib>:"Linear Fit.vi"("Y"=w973, "X"=w972, "method"=w998) -> ("slope"=w986:dbl)  [unwired: 8 in, 4 out]
                                n371 = node(w1036, w1029, "db_insert_data" ("function name"), w1034, w1033, w975, w976, w977, w978, w979, w980, w962, w970, w968, w971, w972, w973) -> (w1032:refnum<k35>, w1031:errorcluster, w1030:refnum<k38>, w983:i32)  [unwired: 13 in, 2 out]
                                n372 = Max & Min(x=w970, y=w992) -> (max(x,y)=w991:dbl)  [unwired: 1 out]
                                n373 = Max & Min(x=w990, y=w970) -> (min(x,y)=w989:dbl)  [unwired: 1 out]
                                n374 = Max & Min(x=w986, y=w988) -> (max(x,y)=w985:dbl)  [unwired: 1 out]
                                n375 = Max & Min(x=w987, y=w986) -> (min(x,y)=w984:dbl)  [unwired: 1 out]
                                n376 = Replace Array Subset(array=w994, new element=w986, index (row)=w979, index (col)=w980) -> (w993:dbl[][])
                                n377 = Replace Array Subset(array=w996, new element=w970, index (row)=w979, index (col)=w980) -> (w995:dbl[][])
                                }
                                n378 = Bundle(w948, w947) -> (→"IZCurve":cluster{dbl[], dbl[]})  [unwired: 1 in]
                                n379 = local write "Pressure Slope Map"(w935) -> ()
                                n380 = local write "Topography"(w936) -> ()
                                }
                                }
                              }
                              frame #2 {
                                n381 = Wait (ms)(milliseconds to wait=u32 50) -> ()  [unwired: 1 out]
                              }
                            }
                          }
                        }
                      }
                    }
                    frame #2 {
                      n382 = Delete Data Value Reference(data value reference=w1397) -> ()  [unwired: 1 in, 2 out]
                      n383 = Release Queue(queue=w1399) -> ()  [unwired: 2 in, 3 out]
                      n384 = node(w1396, w1394, "db_end_frame_timer" ("function name"), w1395, w1391, w1385, w1386, w1387) -> (w1393:refnum<k35>, w1392:errorcluster, w1390:refnum<k38>)  [unwired: 5 in, 2 out]
                    }
                  }
                }
              }
              frame #3 {
                n385 = local read "Adapted_XOffset um"() -> (w1401:dbl)
                n386 = local read "Adapted_YOffset um"() -> (w1400:dbl)
                n387 = local read "Adapted_YNum"() -> (w1404:i32)
                n388 = local read "Adapted_XNum"() -> (w1405:i32)
                n389 = local read "XStepSize um"() -> (w1403:dbl)
                n390 = local read "YStepSize um"() -> (w1402:dbl)
              }
            }
          }
        }
        frame #5 {
          n391 = local read "Retract (edge) um"() -> (w1422:dbl)
          n392 = local read "NF_AppRate um/s"() -> (w1424:dbl)
          n393 = local read "FF_AppRate um/s"() -> (w1423:dbl)
          n394 = node(w1436, w1430, "db_end_global_timer" ("function name"), w1435, w1434) -> (w1433:refnum<k35>, w1432:errorcluster, w1431:refnum<k38>)  [unwired: 2 in, 2 out]
          n395 = local read "Retract (flat) um"() -> (w1425:dbl)
          n396 = local read "FF_Threshold %"() -> (w1427:dbl)
          n397 = local read "NF_Threshold %"() -> (w1426:dbl)
          n398 = local read "Pressure kPa"() -> (w1420:dbl)
          n399 = local read "FrameNum"() -> (w1419:u32)
          n400 = local read "Notes"() -> (w1421:string)
          n401 = node(w1433, w1430, "db_insert_info" ("function name"), w1432, w1431, 0, w1417, w1416, w1415, w1414, w1413, w1412, w1427, w1426, w1425, w1422, w1423, w1424, w1418, w1419, w1420, w1421) -> (w1440:refnum<k35>, w1439:errorcluster, w1438:refnum<k38>)  [unwired: 19 in, 2 out]
          n402 = Close Python Session(session in=w1440, error in=w1439) -> ()  [unwired: 1 out]
          n403 = Close Reference(reference=w1438) -> ()  [unwired: 1 in, 1 out]
        }
        frame #6 {
          n404 = local write "Done?"(TRUE ("Done?")) -> ()
        }
      }
      n405 = while {
        tunnel: w30 -> [w41]
        stop <- w43 stop-if-true
        n406 = local read "Done?"() -> (w44:bool)
        n407 = Or(x="stop", y=w44) -> (x .or. y?=w43:bool)
        n408 = case shown="True" "stop" {
          tunnel: w41 -> [_ w46]
          tunnel: "stop" -> [_ w45]
          frame False {
          }
          frame True {
            n409 = Lossy Enqueue Element(queue=w46, element=w45) -> ()  [unwired: 1 in, 4 out]
          }
        }
        n410 = Wait (ms)(milliseconds to wait=u32 50) -> ()  [unwired: 1 out]
      }
    }
    frame #2 {
      n411 = Release Queue(queue=w1444) -> ()  [unwired: 2 in, 3 out]
    }
  }
